vi "Dashboard Main.vi"() -> ()   [LabVIEW 2020]
uses:
  <vilib>/Utility/miscctls.llb/LVRowAndColumnTypeDef.ctl
  <vilib>/event_ctls.llb/eventvkey.ctl
  2be0e37a-cf1f-4fec-827e-dc22e69ce85b.vi
  77231be5-4dfd-47d5-a2ff-3724d3268e1c.vi
  6c3be22e-c06e-40dd-b218-0ec3cd26438d.vi
  b3ffd77c-c7a0-4f90-8868-8b56e10d7f8c.vi
  67fa5a46-adf3-4589-a2f7-66a250c43ad7.vi
  788908d1-300c-4db3-916d-f2facaeaae96.vi
  e87f41cb-5a92-4aba-b85e-f5fa50e1b7bd.vi
  bca209f3-dc8a-45d9-88b4-0d3b0861506d.vi
  fb4473b5-3a86-49a6-a9b5-0e1129129e81.vi
  849cc23d-0ef3-4264-9ef7-306e991d33d4.vi
  16c4a620-4255-445b-bb5a-a821105b922f.vi
  55761e46-cf36-4bf9-9854-b902932db1d3.vi
  <vilib>/Rock Robotics/Network Tables/NT Write Boolean.vi
  <vilib>/Rock Robotics/Network Tables/NT Read Boolean.vi
  MARS Created VIs/GlobalDataNames.vi
  <vilib>/Rock Robotics/Network Tables/NT Read Boolean Array.vi
  <vilib>/Rock Robotics/Network Tables/NT Read Numeric Array.vi
  <vilib>/Rock Robotics/Network Tables/NT Write Boolean Array.vi
  <vilib>/Rock Robotics/Network Tables/NT Write String Array.vi
  <vilib>/Rock Robotics/Network Tables/NT Write Numeric Array.vi
  <vilib>/Rock Robotics/WPI/Dashboard/WPI_DashboardLogging Global.vi
  <vilib>/Utility/Data Type/NI_Data Type.lvlib
  <vilib>/Utility/Data Type/Type Definitions/Data Type.ctl
panel:
  in  "Camera Settings":T1={"Frame Rate"=15, "Compression"=30, "Size"=1, "DB Camera Config"=TRUE} {"Frame Rate" scale=1.0..30.0; "Compression" scale=100.0..-1.0; "Size" items=["640x480", "320x240", "160x120"]}
  in  "Camera Name":string(combo)="No Camera Selection"
  out "Driver Controls":string[](array[string])=["Teleop-\nPilot-\nleft joystick X & Y axes- swerve strafe / lateral and vertical throttle (field-oriented, based on IMU)\nright joystick X axis- swerve rotational throttle\nLeft trigger- intaking balls\nLeft bumper- outtake balls\nRight trigger- fire shooter\nRight bumper- puke ball\nY button- zero pose (IMU & odometry, the odometry zeroes to touching the right post of our team’s launch pad)\nB button- disable turret safety\n\nCo-pilot-\nleft joystick X & Y- control turret field-based\nleft joystick push- change turret control to be %vbus \nright joystick Y- outer arm elevator\nleft/right bumper- inner arm pivot back/forward respectfully\nleft/right triggers- outer arm pivot back/vertical respectfully\nX button- move turret and cowl to zero\nY button- toggle climber sequence\nA button- confirm step advance\nB button- toggle always-tracking turret & passive flywheel (off by default)\nD-pad Up/Down- run magazine forwards/backwards respectfully\nD-pad right/left- run funnel forwards/backwards respectfully\n\n*the manual climb pneumatic controls only override the climb sequence when the buttons are held down. once released, the pneumatic goes back to the state it was at previously*", "Test Controls:\nPilot-\nleft joystick X & Y axes- swerve strafe / lateral and vertical throttle (robot-oriented)\nright joystick X axis- swerve rotational throttle\nA button- toggle intake pneumatic\nleft trigger- run intake motor\nRight trigger- run flywheel\nD-pad Up/Down- run magazine forwards/backwards respectfully\nD-pad right/left- run funnel forwards/backwards respectfully\nB button (hold)- disable limits on outer arm pivot, outer arm elevator, inner arm pivot, turret, and cowl\nX button- set new zero values to the current spots on those ^\nY button- zero pose (IMU & odometry)\n\nCopilot-\nleft joystick X- control turret\nright joystick Y- outer arm elevator\nleft/right bumper- inner arm pivot back/forward respectfully\nleft/right triggers- outer arm pivot back/vertical respectfully\nView/Menu button- move cowl down/up respectfully\nY button- toggle climber sequence\nA button- confirm step advance\n", "LED Colors-\nnormal\t\t\t\tred\ntargeting... \t\t\tyellow\nfiring! \t\t\t\tgreen\nno target seen\t\t\tblue\nball in magazine\t\torange\nclimb sequence started \tpurple\nclimb step finished\t\twhite\nauto is happening\t\tpink\nauto play ended\t\tbeige\n"]
  in  "TCP":refnum<k5>
  out "Robot IP":string="0.0.0.0"
  out "Image Message":string="Timeout in Camera Communications"
  in  "Dashboard Tab":T2(tab)
  in  "SWM_LL_Threshold (in)":dbl=143.0
  in  "SWM_Magnitude_Limit":dbl=0.3
  in  "SWM_Moving_Threshold (ft/s)":dbl=0.1
  in  "Turret_Max_Offset(deg)":dbl=2.0
  in  "Turret_Offset":dbl=2.0
  out "BR_Zero":dbl
  out "BR_Position":dbl
  out "BL_Zero":dbl
  out "BL_Position":dbl
  out "FL_Zero":dbl
  out "FL_Position":dbl
  out "FR_Zero":dbl
  out "FR_Position":dbl
  in  "Max_Ground_Speed(ft/s)":dbl
  in  "Cowl_Kp":dbl=0.06
  in  "Manual_Magazine_Power":dbl=0.4
  in  "Flywheel_Speed_Multiplier":dbl=1.0
  in  "Flywheel_Acceptable_Error":dbl=200.0
  in  "Turret_Upper_Limit_Value":dbl=160.0
  in  "Turret_Lower_Limit_Value":dbl=-160.0
  in  "Turret_Kd":dbl=0.001
  in  "Turret_Ki":dbl=1e-05
  in  "Turret_Kp":dbl=0.06
  in  "BL_Min Output":dbl=-0.5 min=0.0
  in  "BR_Max Ouput":dbl=0.5 min=0.0
  in  "BR_Int Error Window":dbl=20.0 min=0.0
  in  "BR_N-Int":i32=10 min=0
  in  "BR_N-Diff":i32=10 min=0
  in  "BR_Kd":dbl min=0.0
  in  "BR_Ki":dbl min=0.0
  in  "BR_Kp":dbl=0.0028 min=0.0
  in  "BL_Min Output":dbl=-0.5 min=0.0
  in  "BL_Max Ouput":dbl=0.5 min=0.0
  in  "BL_Int Error Window":dbl=20.0 min=0.0
  in  "BL_N-Int":i32=10 min=0
  in  "BL_N-Diff":i32=10 min=0
  in  "BL_Kd":dbl min=0.0
  in  "BL_Ki":dbl min=0.0
  in  "BL_Kp":dbl=0.0028 min=0.0
  in  "FL_Min Output":dbl=-0.5 min=0.0
  in  "FL_Max Ouput":dbl=0.5 min=0.0
  in  "FL_Int Error Window":dbl=20.0 min=0.0
  in  "FL_N-Int":i32=10 caption="FR_N-Int" min=0
  in  "FL_N-Diff":i32=10 min=0
  in  "FL_Kd":dbl min=0.0
  in  "FL_Ki":dbl min=0.0
  in  "FL_Kp":dbl=0.0028 min=0.0
  in  "FR_Min Output":dbl=-0.5 min=0.0
  in  "FR_Max Ouput":dbl=0.5 min=0.0
  in  "FR_Int Error Window":dbl=20.0 min=0.0
  in  "FR_N-Int":i32=10 min=0
  in  "FR_N-Diff":i32=10 min=0
  in  "FR_Kd":dbl min=0.0
  in  "FR_Ki":dbl min=0.0
  in  "FR_Kp":dbl=0.0028 min=0.0
  out "Cowl_Position(Degrees)":dbl(knob)=45.0 scale=-180.0..180.0
  out "Orientation_State":enum16{"Robot-Oriented", "Field-Oriented"}(ring)
  out "Back_Right_Drive_Command":dbl(slide) scale=0.0..1.0 scale format="%.2f"
  out "Back_Right_Angle_Command(deg)":dbl(knob) scale=180.0..-180.0 scale format="%#_6f"
  out "Back_Left_Drive_Command":dbl(slide) scale=0.0..1.0 scale format="%.2f"
  out "Back_Left_Angle_Command(deg)":dbl(knob) scale=180.0..-180.0 scale format="%#_6f"
  out "Front_Left_Drive_Command":dbl(slide) scale=0.0..1.0 scale format="%.2f"
  out "Front_Left_Angle_Command(deg)":dbl(knob) scale=180.0..-180.0 scale format="%#_6f"
  out "Front_Right_Drive_Command":dbl(slide) scale=0.0..1.0 scale format="%.2f"
  out "Front_Right_Angle_Command(deg)":dbl(knob) scale=180.0..-180.0 scale format="%#_6f"
  out "Flywheel_Velocity(RPM)":dbl(slide)=2614.0 scale=0.0..5000.0 scale format="%#_5g"
  out "Turret_Absolute_Position(Degrees)":dbl(knob)=45.0 scale=-180.0..180.0
  out "Camera Image":T3(plugin-control)
  out "Camera Perf":string="                          "
  out "Magazine_Velocity":dbl
  out "BoolTableSize":i32
  out "NumTableSize":i32
  out "StrTableSize":i32
  out "Selector":string="Initialize"
  out "NTEmpty":bool=TRUE
  out "disconnected":bool=TRUE
  out "ValuesGotOverwritten":bool
  in  "Select Auto":string(combo)="Select Autonomous ..."
  out "NT Connection":bool
  out "JS1 Z":dbl(slide) scale=-1.0..1.0 scale format="%#_2e"
  out "JS1 Graph":cluster{"X":dbl, "Y":dbl}[](graph)
  out "JS1 Buttons":T4
  out "JS2 Z":dbl(slide) scale=-1.0..1.0 scale format="%#_2e"
  out "JS2 Graph":cluster{"X":dbl, "Y":dbl}[](graph)
  out "JS2 Buttons":T4
  out "Mode":T5(ring)=enum."Disconnected"
  out "Right Camera Perf":cluster{"Bandwidth (Mbps)":dbl, "FPS":dbl}
  out "Camera Image Right":T3(plugin-control)
  in  "Camera Settings Right":T1={"Frame Rate"=15, "Compression"=30, "Size"=1, "DB Camera Config"=FALSE} {"Frame Rate" scale=1.0..30.0; "Compression" scale=100.0..-1.0; "Size" items=["640x480", "320x240", "160x120"]}
  in  "Camera Name Right":string(combo)="No Camera Selection"
  in  "Rec Mode":enum32{"Stop", "Record", "Playback"}(radio)
  in  "DB/String 9":string
  in  "DB/String 8":string
  in  "DB/String 7":string
  in  "DB/String 6":string
  in  "DB/String 5":string
  in  "DB/String 4":string
  in  "DB/String 3":string
  in  "DB/String 2":string
  in  "DB/String 1":string
  in  "DB/String 0":string
  in  "DB/Slider 0":dbl(slide) scale=0.0..5.0
  in  "DB/Slider 1":dbl(slide) scale=0.0..5.0
  in  "DB/Slider 2":dbl(slide) scale=0.0..5.0
  in  "DB/Slider 3":dbl(slide) scale=0.0..5.0
  out "DB/LED 3":bool
  out "DB/LED 2":bool
  out "DB/LED 1":bool
  out "DB/LED 0":bool
  in  "DB/Button 3":bool
  in  "DB/Button 2":bool
  in  "DB/Button 1":bool
  in  "DB/Button 0":bool caption="New Name"
  in  "Test Slider":dbl(slide) scale=0.0..100.0 scale format="%#_3g"
  in  "On/Off":bool caption="Solenoid"
  in  "Test Name":u16(ring) items=["Select the test to run..."]
  in  "Test Tree":string(tree)
  in  "Motor":cluster{"Value":dbl, "Enable":bool} {"Value" scale=-1.0..1.0 scale format="%#_3g"}
  out "Progress":T6 {"Test Progress" scale=0.0..100.0}
  in  "Rev/Fwd":cluster{"Forward":bool, "Reverse":bool}
  in  "Test Ring":u16(ring) items=["Monochrome", "Color"]
  out "Cmd Status":string
  in  "Execute Command":bool
  in  "Command Params":string[][](table)
  in  "Command Selection":i32(listbox)
  in  "CheckList":i32(listbox)
  out "Tree":string(tree)
  out "SWM_In_Range":bool
  in  "Alpha_Limelight_Mounting_Angle(deg)":dbl=35.0
  out "Limelight_Distance_To_Target (in)":dbl
  in  "Zero_Swerves":bool
  in  "Funnel_Load_%Vbus":dbl=0.7
  in  "Magazine_Load_%Vbus":dbl=0.3
  in  "Intake_Load_%Vbus":dbl=0.5
  out "Drive_IMU_Yaw":dbl
  out "Robot_Y":dbl
  out "Robot_X":dbl
  out "Limelight_Disconnected":bool
  out "Flywheel_Spun_Up":bool
  out "Turret_Locked":bool
  out "Camera Image 2":T3(plugin-control)
  in  "Auto_Play_Selector":string(combo)="A-No-Op"
  in  "Magazine_Firing_Velocity":dbl=6300.0
  out "Background":bool
  # "0- Teleop 1- Test 2- LED"
  # "HW"
  # "Funnel"
  # "Turret"
  # "Cowl"
  # "Flywheel"
  # "Constant"
  # "Magazine"
  # "Shooting While Moving"
  # "Drive"
  # "Drive Commands"
  # "Front_Left"
  # "Front_Right"
  # "Back_Left"
  # "Back_Right"
  # "Joysticks"
  # "Drive Motors"
  # "Front"
  # "Right"
  # "Left"
  # "Back"
  # "HW"
  # "This tab is a great place for autonomous settings and robot-specific values.\nPlace controls and indicators inside this tab and match name to\nDashboard Variables on robot. You can also delete this comment."
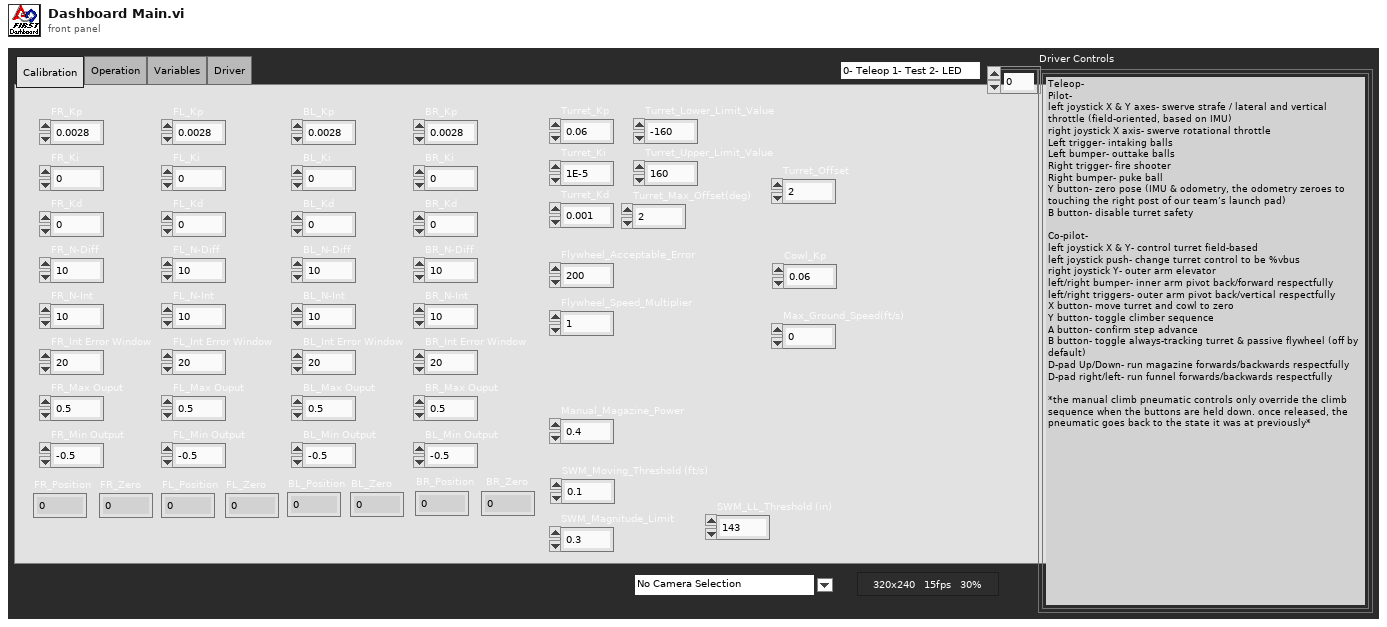
[diagram p1: front panel]
types:
  T1 = cluster{"Frame Rate":i32, "Compression":i32, "Size":u16, "DB Camera Config":bool}
  T2 = enum32{"Calibration", "Operation", "Testing", "Drive", "Camera", "Basic", "Custom", "Test", "Commands", "Checklist", "Variables", "Driver"}
  T3 = typedef "IMAQ Image.ctl" = refnum<image>
  T4 = cluster{bool, bool, bool, bool, bool, bool, bool, bool, bool, bool, bool, bool}
  T5 = enum8{"Tele-Op Disabled", "Tele-Op Enabled", "Auto Disabled", "Auto Enabled", "Test Disabled", "Test Enabled", "Disconnected", "No Code", "E-Stop"}
  T6 = cluster{"Test Progress":u8, "Test Progress Text":string}
  T7 = cluster{"Save Path":path, "Interval (s)":dbl, "Keep":i32}
  T8 = typedef "Image Type" = u32
  T9 = cluster{"IDs":cluster{"RPC field ID":u16, "Unique ID":u16}, "String":string}
  T10 = cluster{"Error Strings":string, "Disable Counts":cluster{u16, u16}, "Rail Faults":cluster{u16, u16, u16}, "Robot IP":string, "DB Mode":u8, "Event Info":cluster{"Name":string, "Type":u8, "Number":u16, "Replay":u8}}
  T11 = cluster{"Storage":cluster{"Disk Free":u64, "RAM Block":u32, "RAM free":u32}, "CPU Utilization":cluster{"CPU % ISR":sgl, "CPU % Time Crit":sgl, "CPU % Timed Str":sgl, "CPU % High":sgl, "CPU % Above":sgl, "CPU % Normal":sgl, "CPU % Low":sgl}, "CAN":cluster{"% Bus Utilization":sgl, "Bus Off Cnt":u32, "TX_FIFO Full Cnt":u32, "Receive Error Cnt":u8, "Transmit Error Cnt":u8}, "HID":cluster{"HID Outputs":u32, "Rumble Low":u16, "Rumble High":u16}[]}
  T12 = cluster{"Status bits":cluster{"Test Mode":bool, "Autonomous":bool, "Enabled":bool, "Code Start":bool, "Brownout":bool, "Reserved 2":bool, "Reserved 3":bool, "E-Stop":bool}, "Code Trace":cluster{"Disabled":bool, "TeleOp":bool, "Auto":bool, "Test":bool}, "Controller Type":enum16{"unknown", "cRIO", "roboRio"}, "Code?":enum16{"unknown", "noCode", "code"}, "Battery V":dbl}
  T13 = cluster{"Control Bits":cluster{"TestMode":bool, "Autonomous":bool, "Enabled":bool, "FMS Present":bool, bool, bool, bool, "E-Stop":bool}, "Team Station ":u8, "Countdown":sgl, "Joystick Values":cluster{"Axes":dbl[], "Buttons":bool[], "POVs":i16[]}[]}
  T14 = cluster{"Axes":dbl[], "Buttons":bool[], "POVs":i16[]}[]
  T15 = cluster{"Axes":dbl[], "Buttons":bool[], "POVs":i16[]}
  T16 = cluster{"Buttons[0]":bool, "Buttons[1]":bool, "Buttons[2]":bool, "Buttons[3]":bool, "Buttons[4]":bool, "Buttons[5]":bool, "Buttons[6]":bool, "Buttons[7]":bool, "Buttons[8]":bool, "Buttons[9]":bool, "Buttons[10]":bool, "Buttons[11]":bool}
  T17 = cluster{"Camera Image":refnum<vi>, "Dashboard Tab":refnum<vi>, "Background":refnum<vi>, "Rec Mode":refnum<vi>, "Test Slider":refnum<vi>, "On/Off ":refnum<vi>, "Test Ring":refnum<vi>, "Rev/Fwd":refnum<vi>, "Test Name":refnum<vi>, "Motor":refnum<vi>, "Progress":refnum<vi>, "CheckList":refnum<vi>, "Tree":refnum<vi>, "Test Tree":refnum<vi>, "Command Params":refnum<vi>, "Command Selection":refnum<vi>, "Execute Command":refnum<vi>, "Cmd Status":refnum<vi>, "Camera Settings":refnum<vi>, "Camera Name":refnum<vi>, "Camera Perf":refnum<vi>, "Camera Settings Right":refnum<vi>, "Camera Name Right":refnum<vi>, "Camera Image Right":refnum<vi>}
  T18 = cluster{"Global Rectangle":i32[], "Contours":cluster{"Contour Type":u32, "ROI Type":u32, "Points":i32[]}[]}
  T19 = cluster{"Camera Name":string, string, "Saved DB Images Info":cluster{"Save Path":path, "Interval (s)":dbl, "Keep":i32}}
  T20 = cluster{"Camera Name Right":string, string, "Saved DB Images Info":cluster{"Save Path":path, "Interval (s)":dbl, "Keep":i32}}
  T21 = cluster{"Operation":enum16{"Update", "Clear"}, "Color Box":u32}[]
  T22 = typedef "eventvkey.ctl" = enum16{"ASCII", "Enter", "Return", "Shift", "Ctrl", "Alt", "Cmd", "Opt", "Caps", "NumLock", "Clear", "Break", "Up", "Down", "Left", "Right", "Insert", "Delete", "Home", "End", "PageUp", "PageDown", "Escape", "Help", "Pause", "ScrollLock", "F1", "F2", "F3", "F4", "F5", "F6", "F7", "F8", "F9", "F10", "F11", "F12", "F13", "F14", "F15", "F16", "F17", "F18", "F19", "F20", "F21", "F22", "F23", "F24", "Play", "VolumeUp", "VolumeDown", "Mute", "Two Byte Char"}
  T23 = cluster{"Image Size":bool, "Image Type":bool, "Pixel Value":bool, "ROI Information":bool, "Zoom Factor":bool}
  T24 = cluster{"Operation":enum16{"Update", "Clear"}, "Color Box":u32}
  T25 = typedef "LVRowAndColumnTypeDef.ctl" = cluster{"Row":i32, "Column":i32}
  T26 = cluster{"Shift":bool, "Ctrl":bool, "Alt":bool, "Cmd":bool, "Opt":bool}
  T27 = typedef "NI_Data Type.lvlib/Data Type.ctl" = enum8{"Invalid Type", "Void", "I8", "I16", "I32", "I64", "U8", "U16", "U32", "U64", "Single Float", "Double Float", "Extended Float", "Single Complex", "Double Complex", "Extended Complex", "Enum U8", "Enum U16", "Enum U32", "Enum U64", "Single Float With Unit", "Double Float With Unit", "Extended Float With Unit", "Single Complex with Unit", "Double Complex with Unit", "Extended Complex with Unit", "Boolean", "String", "Path", "Picture", "Tag", "Array", "Cluster", "Variant", "LV Variant", "Waveform", "Timestamp", "Digital Waveform", "Digital Data", "ExpressData", "Refnum", "External Data", "VI", "Poly VI", "LabVIEW Class Instance", "Fixed Point", "Set Collection", "Map Collection"}
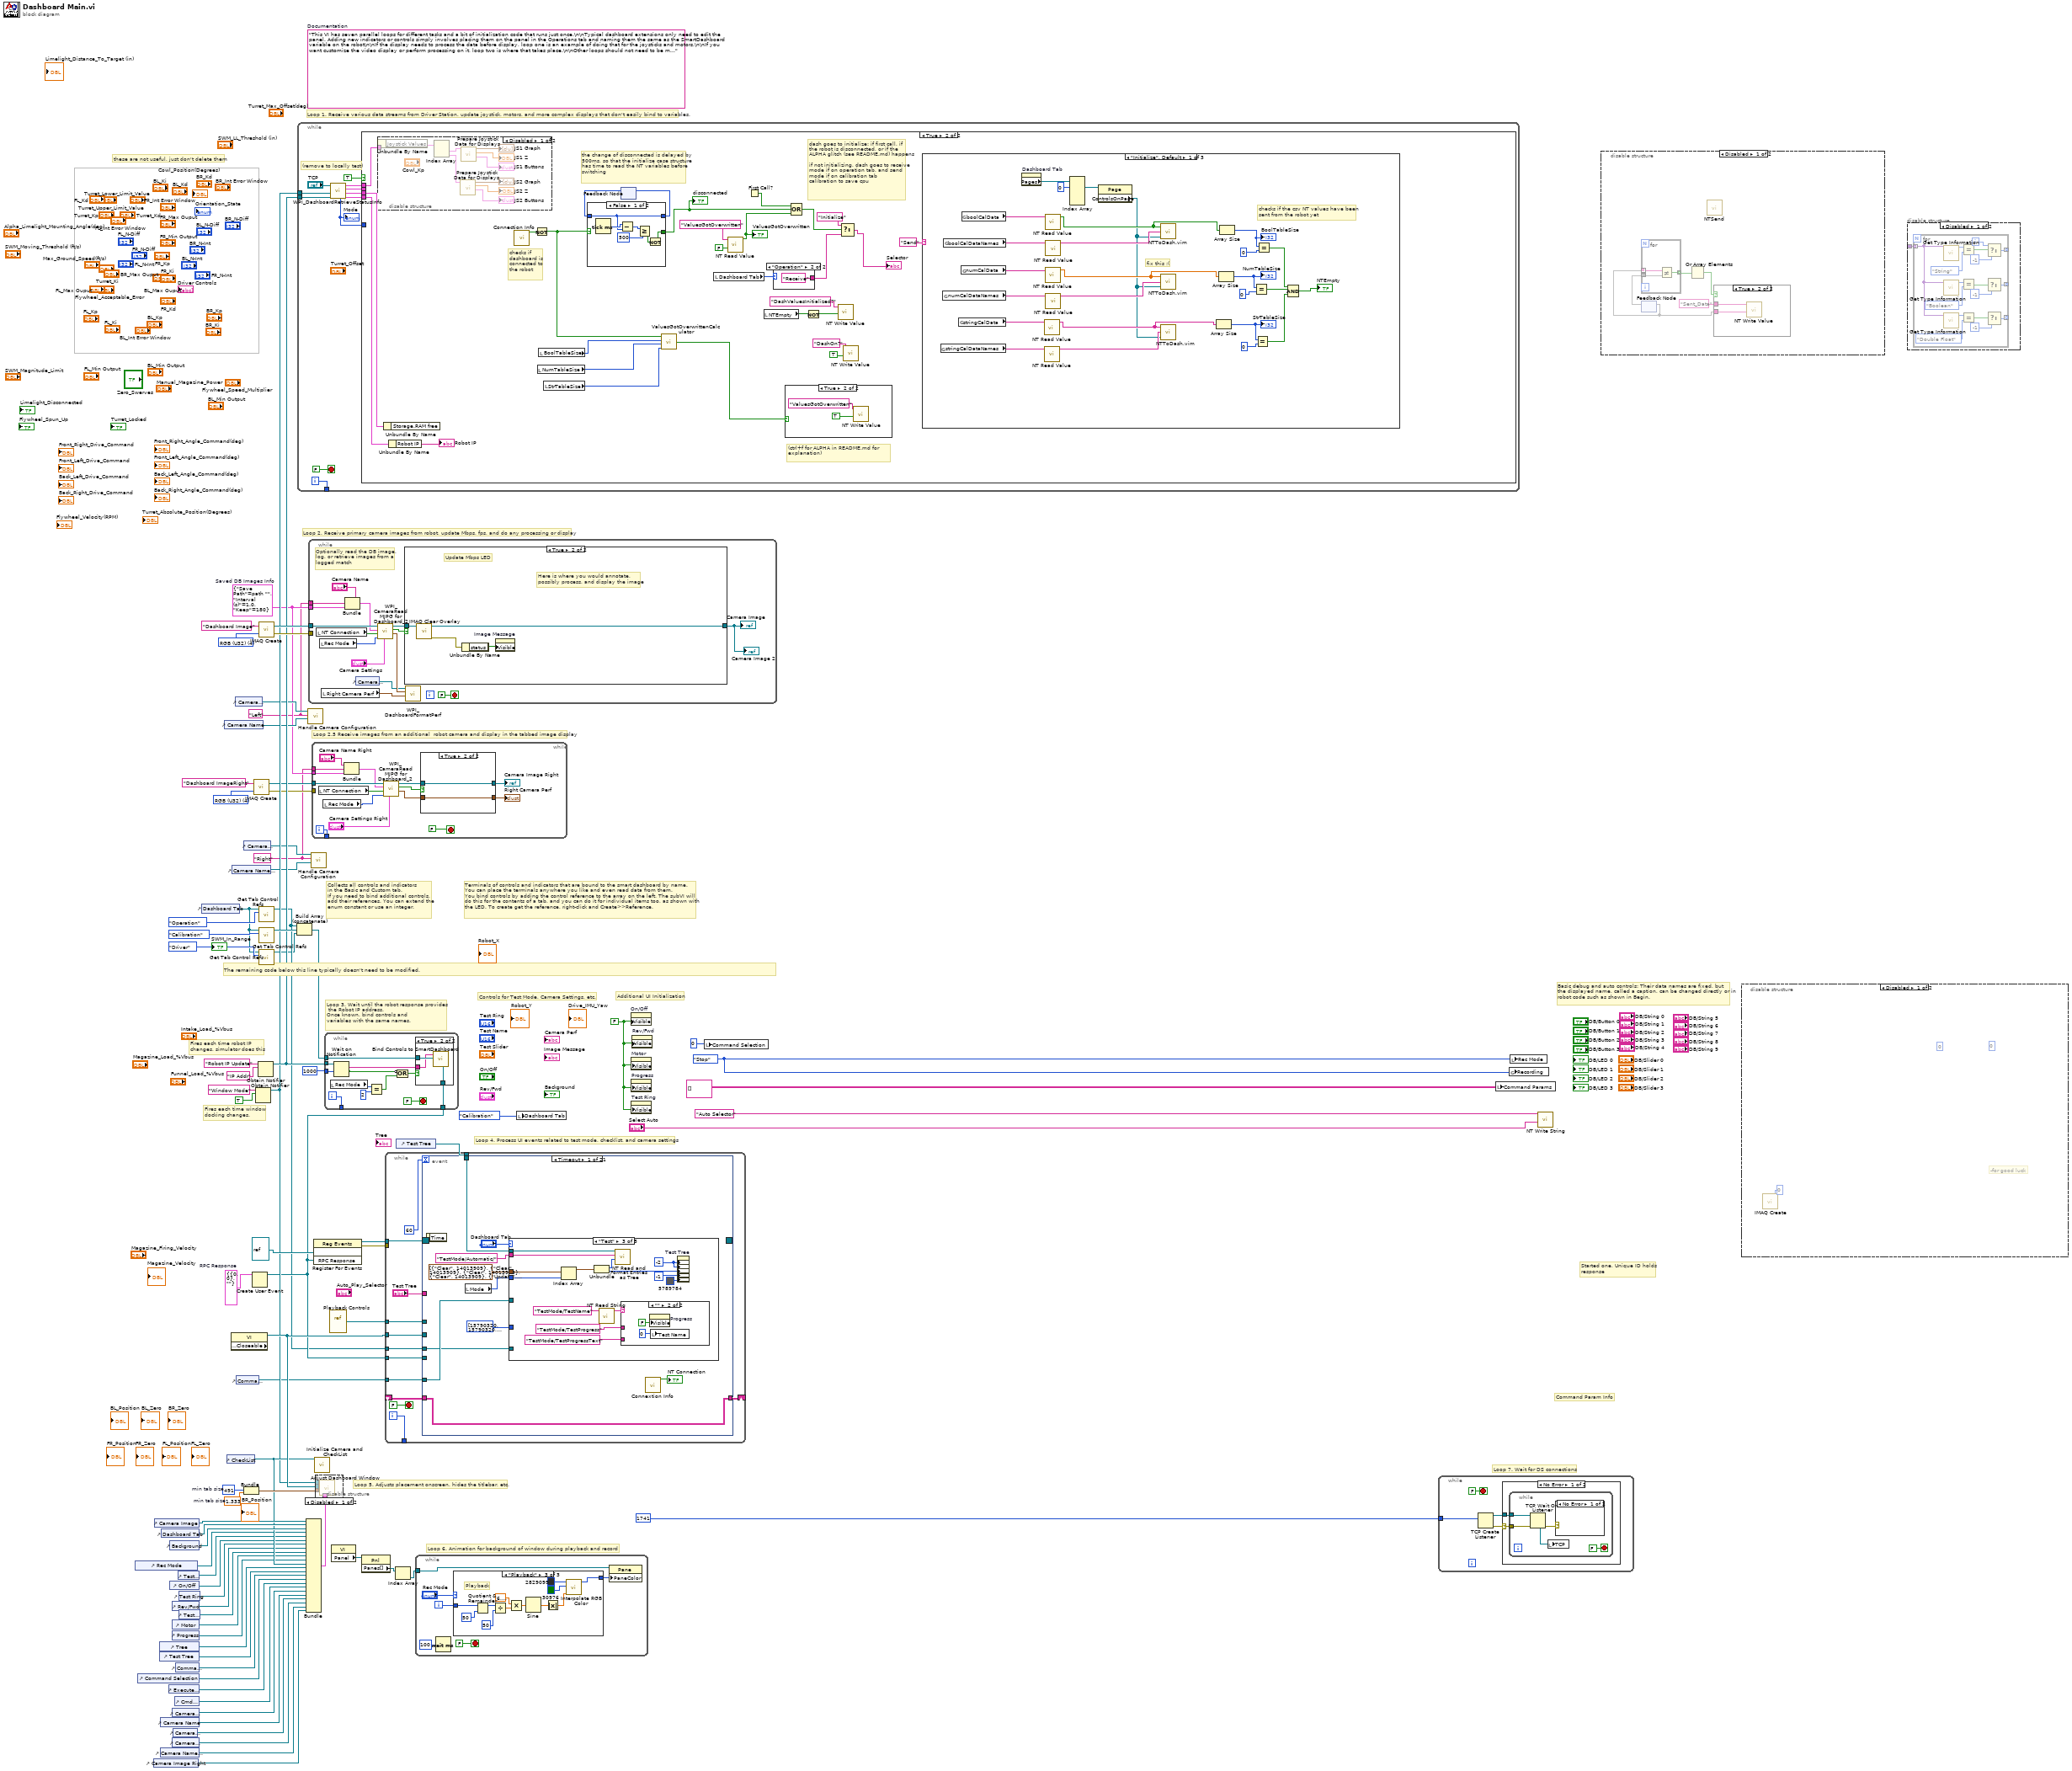
[diagram p0: block diagram]
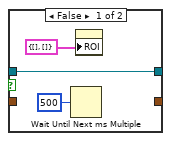
[diagram p7: hidden frame]
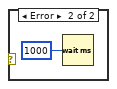
[diagram p8: hidden frame]
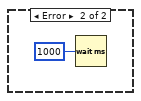
[diagram p9: hidden frame]
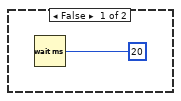
[diagram p10: hidden frame]
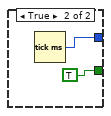
[diagram p12: hidden frame]
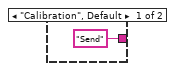
[diagram p14: hidden frame]
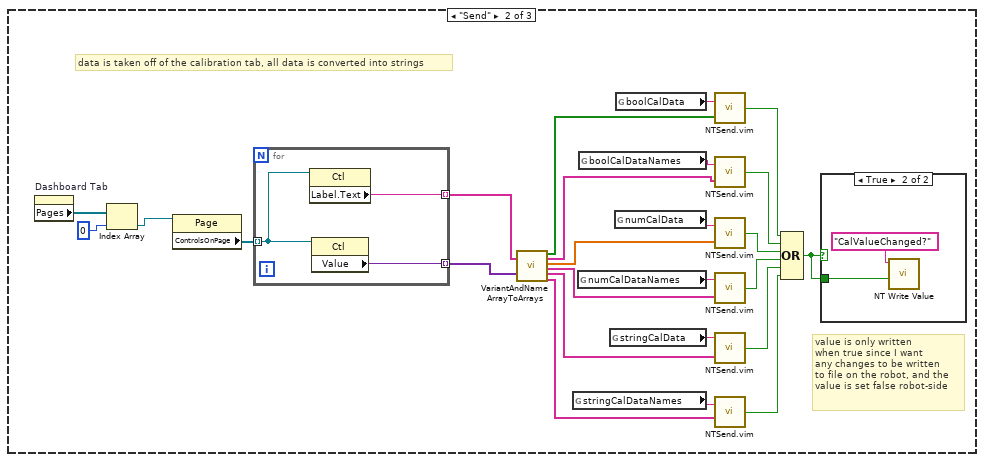
[diagram p15: hidden frame]
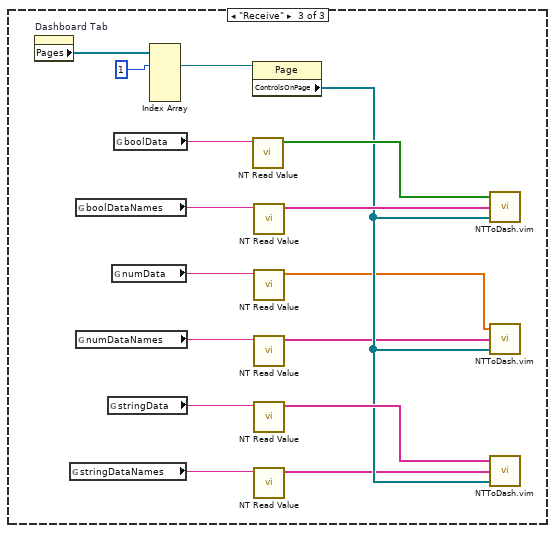
[diagram p17: hidden frame]
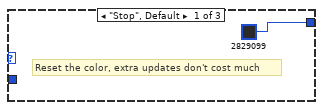
[diagram p18: hidden frame]
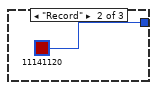
[diagram p19: hidden frame]
diagram:
  w9 = T7 {"Save Path"=path "", "Interval (s)"=1.0, "Keep"=180}  # Saved DB Images Info
  w8 = "Right"
  w7 = "Left"
  w17 = T8 4 items=["Grayscale (U8)", "Grayscale (I16)", "Grayscale (SGL)", "Complex (CSG)", "RGB (U32)", "HSL (U32)", "RGB (U64)"] ("Image Type")
  w33 = T9 {"IDs"={"RPC field ID"=0, "Unique ID"=0}, "String"=""}  # RPC Response
  w55 = 491  # min tab size
  w54 = 1.333  # min tab size
  w61 = enum32{"Stop", "Record", "Playback"}."Stop" ("Rec Mode")
  w39 = FALSE ("Visible")
  (unwired) "This VI has seven parallel loops for different tasks and a bit of initialization code that runs just once.\n\nTypical dashboard extensions only need to edit the panel. Adding new indicators or controls simply involves placing them on the panel in the Operations tab and naming them the same as the SmartDashboard variable on the robot\n\nIf the display needs to process the data before display, loop one is an example of doing that for the joysticks and motors.\n\nIf you want customize the video display or perform processing on it, loop two is where that takes place.\n\nOther loops should not need to be modified. They are pretty standard, and document the task they perform."  # Documentation
  w78 = T8 4 items=["Grayscale (U8)", "Grayscale (I16)", "Grayscale (SGL)", "Complex (CSG)", "RGB (U32)", "HSL (U32)", "RGB (U64)"] ("Image Type")
  # "these are not useful, just don't delete them"
  # "Loop 2.5 Receive images from an additional  robot camera and display in the tabbed image display"
  # "Command Param Info"
  # "Started one, Unique ID holds\nresponse"
  # "Loop 7. Wait for DS connections"
  # "Basic debug and auto controls: Their data names are fixed, but\nthe displayed name, called a caption, can be changed directly or in\nrobot code such as shown in Begin."
  # "Controls for Test Mode, Camera Settings, etc."
  # "Additional UI Initialization"
  # "Loop 6. Animation for background of window during playback and record"
  # "Fires each time robot IP\nchanges, simulator does this"
  # "Fires each time window\ndocking changes."
  # "Collects all controls and indicators\nin the Basic and Custom tab.\nIf you need to bind additional controls,\nadd their references. You can extend the\nenum constant or use an integer."
  # "The remaining code below this line typically doesn't need to be modified."
  # "Loop 4. Process UI events related to test mode, checklist, and camera settings"
  # "Terminals of controls and indicators that are bound to the smart dashboard by name.\nYou can place the terminals anywhere you like and even read data from them.\nYou bind controls by adding the control reference to the array on the left. The subVI will\ndo this for the contents of a tab, and you can do it for individual items too, as shown with\nthe LED. To create get the reference, right-click and Create>>Reference."
  # "Loop 3. Wait until the robot response provides\n the Robot IP address.\nOnce known, bind controls and\nvariables with the same names."
  # "Loop 5. Adjusts placement onscreen, hides the titlebar, etc."
  # "Loop 1. Receive various data streams from Driver Station, update joystick, motors, and more complex displays that don't easily bind to variables."
  # "Loop 2. Receive primary camera images from robot, update Mbps, fps, and do any processing or display"
  n1 = control-ref of="Rec Mode"() -> (w45:refnum<vi>)
  n2 = control-ref of="Command Selection"() -> (w32:refnum<vi>)
  n3 = control-ref of="Camera Image Right"() -> (w10:refnum<vi>)
  n4 = control-ref of="Camera Image"() -> (w57:refnum<vi>)
  n5 = control-ref of="Tree"() -> (w49:refnum<vi>)
  n6 = control-ref of="Test Tree"() -> (w48:refnum<vi>)
  n7 = control-ref of="Camera Name"() -> (w23:refnum<vi>)
  n8 = control-ref of="Camera Name Right"() -> (w11:refnum<vi>)
  n9 = control-ref of="Dashboard Tab"() -> (w56:refnum<vi>)
  n10 = control-ref of="Execute Command"() -> (w34:refnum<vi>)
  n11 = control-ref of="Background"() -> (w52:refnum<vi>)
  n12 = control-ref of="On/Off"() -> (w43:refnum<vi>)
  n13 = control-ref of="Progress"() -> (w40:refnum<vi>)
  n14 = control-ref of="Camera Settings"() -> (w24:refnum<vi>)
  n15 = control-ref of="Camera Settings Right"() -> (w12:refnum<vi>)
  n16 = control-ref of="Rev/Fwd"() -> (w41:refnum<vi>)
  n17 = control-ref of="Motor"() -> (w46:refnum<vi>)
  n18 = control-ref of="Camera Perf"() -> (w22:refnum<vi>)
  n19 = control-ref of="Cmd Status"() -> (w28:refnum<vi>)
  n20 = control-ref of="Command Params"() -> (w35:refnum<vi>)
  n21 = control-ref of="Test Slider"() -> (w44:refnum<vi>)
  n22 = control-ref of="Test Ring"() -> (w42:refnum<vi>)
  n23 = control-ref of="Test Name"() -> (w47:refnum<vi>)
  n24 = control-ref of="Dashboard Tab"() -> (w2:refnum<vi>)
  n25 = control-ref of="Camera Name"() -> (w25:refnum<vi>)
  n26 = control-ref of="CheckList"() -> (w50:refnum<vi>)
  n27 = property class="VI" props=["Front Panel.Closeable"]() -> (reference out=w60:refnum<vi>)  [unwired: 2 in, 2 out]
  n28 = control-ref of="Camera Name Right"() -> (w13:refnum<vi>)
  n29 = control-ref of="Camera Settings"() -> (w26:refnum<vi>)
  n30 = control-ref of="Command Params"() -> (w27:refnum<vi>)
  n31 = control-ref of="Camera Settings Right"() -> (w14:refnum<vi>)
  n32 = Bundle("min tab size"=w55, "min tab size"=w54) -> (w53:cluster{"min tab size":i32, "min tab size":dbl})  [unwired: 1 in]
  n33 = Create User Event(user event datatype=w33) -> (user event=w29:refnum<user-event>)  [unwired: 1 in, 1 out]
  n34 = call "IMAQ Create"("Image Name"="Dashboard ImageRight", "Image Type"=w17) -> ("New Image"=w16:T3, "error out"=w15:errorcluster)  [unwired: 2 in, 1 out]
  n35 = Obtain Notifier(name (unnamed)="Window Mode", notification data type=TRUE) -> (notifier out=w37:refnum<notifier>)  [unwired: 2 in, 2 out]
  n36 = Obtain Notifier(name (unnamed)="Robot IP Update", notification data type="IP Addr" ("name (unnamed)")) -> (notifier out=w38:refnum<notifier>)  [unwired: 2 in, 2 out]
  n37 = call "IMAQ Create"("Image Name"="Dashboard Image", "Image Type"=w78) -> ("New Image"=w76:T3, "error out"=w75:errorcluster)  [unwired: 2 in, 1 out]
  n38 = call <vilib>:"Get Tab Control Refs.vi"("Page Index"=T2."Operation" ("Dashboard Tab"), "TabControl in"=w2) -> ("ControlsOnPage"=w21:refnum<vi>[])  [unwired: 9 in]
  n39 = call <vilib>:"Get Tab Control Refs.vi"("Page Index"=T2."Calibration" ("Dashboard Tab"), "TabControl in"=w2) -> ("ControlsOnPage"=w59:refnum<vi>[])  [unwired: 9 in]
  n40 = call <vilib>:"Get Tab Control Refs.vi"("Page Index"=T2."Driver" ("Dashboard Tab"), "TabControl in"=w2) -> ("ControlsOnPage"=w4:refnum<vi>[])  [unwired: 9 in]
  n41 = Build Array (concatenate)(w21, w59, w4) -> (w58:refnum<vi>[])
  n42 = while {
    tunnel: [w88] -> _
    tunnel: w38 -> [w83]
    tunnel: w37 -> [w80]
    i -> [w88]
    stop <- FALSE stop-if-true
    # "(remove to locally test)"
    n43 = call <vilib>:"WPI_DashboardRetrieveStatusInfo.vi"("Binding Refnum"=w83, "Window Mode Notifier"=w80, "TCP Cnx"="TCP") -> ("Power and Errors"=w84:T10, "Robot Metrics"=w86:T11, "Status Info"=w87:T12, "Control Info"=w85:T13, "Robot Mode"=w82:T5)  [unwired: 3 in, 1 out]
    "Mode" <- w82
    n44 = case shown="True" TRUE {
      tunnel: w87 -> [_ _]
      tunnel: w86 -> [_ w118]
      tunnel: w85 -> [_ w117]
      tunnel: w84 -> [_ w116]
      tunnel: w82 -> [_ _]
      frame False {
        n45 = Wait (ms)(milliseconds to wait=u32 20) -> ()  [unwired: 1 out]
      }
      frame True {
        # "checks if dashboard is connected to the robot"
        # "(ctrl+f for ALPHA in README.md for explanation)"
        # "the change of disconnected is delayed by 500ms, so that the initialize case structure has time to read the NT variables before switching"
        # "dash goes to initialize: if first call, if\nthe robot is disconnected, or if the ALPHA glitch (see README.md) happens\n\nif not initializing, dash goes to receive mode if on operation tab, and send mode if on calibration tab\ncalibration to save cpu"
        n46 = disable-structure shown="Disabled" {
          disable-tunnel: w117 -> [w138 _]
          frame Disabled {
            n47 = Unbundle By Name(w138) -> ("Joystick Values"=w137:T14)
            n48 = Index Array(array=w137) -> (element #1=w136:T15, element #2=w132:T15)  [unwired: 2 in]
            n49 = call "Prepare Joystick Data for Displays.vi"("Joystick Values"=w132) -> ("Buttons"=→"JS2 Buttons":T16, "Z Axis"=→"JS2 Z":dbl, "Cartesian Data"=→"JS2 Graph":cluster{"X axis":dbl, "X axis":dbl}[])  [unwired: 8 in]
            n50 = call "Prepare Joystick Data for Displays.vi"("Joystick Values"=w136) -> ("Buttons"=→"JS1 Buttons":T16, "Z Axis"=→"JS1 Z":dbl, "Cartesian Data"=→"JS1 Graph":cluster{"X axis":dbl, "X axis":dbl}[])  [unwired: 8 in]
          }
          frame Enabled {
          }
        }
        n51 = Unbundle By Name(w118) -> ()  [unwired: 1 out]
        n52 = Unbundle By Name(w116) -> ("Robot IP"=→"Robot IP":string)
        n53 = call <vilib>:"Connection Info.vi"() -> ("Connected"=w104:bool)  [unwired: 10 in, 1 out]
        n54 = Not(x=w104) -> (.not. x?=w97:bool)
        n55 = local read "NumTableSize"() -> (w99:i32)
        n56 = local read "BoolTableSize"() -> (w100:i32)
        n57 = local read "StrTableSize"() -> (w98:i32)
        n58 = feedback #1() -> (w101:u32)  [unwired: 1 in]
        n59 = case shown="False" w97 {
          tunnel: [w121 TRUE] -> w103
          tunnel: [w125 w127] -> w102
          tunnel: w101 -> [w125 _]
          frame False {
            n60 = Tick Count (ms)() -> (millisecond timer value=w126:u32)
            n61 = Subtract(x=w126, y=w125) -> (x-y=w124:u32)
            n62 = Greater Or Equal?(x=w124, y=u32 500) -> (x >= y?=w122:bool)
            n63 = Not(x=w122) -> (.not. x?=w121:bool)
          }
          frame True {
            n64 = Tick Count (ms)() -> (millisecond timer value=w127:u32)
          }
        }
        "disconnected" <- w103
        n65 = feedback-in #1(w102) -> ()
        n66 = call "ValuesGotOverwrittenCalculator.vi"("StrTableSize"=w98, "NumTableSize"=w99, "BoolTableSize"=w100, "disconnected"=w97) -> ("ValuesGotOverwritten"=w96:bool)
        n67 = local read "Dashboard Tab"() -> (w112:T2)
        n68 = call-poly <vilib>:"NT Read Value.vi"("Default Value"=FALSE, "Name"="ValuesGotOverwritten") -> ("Boolean"=w93:bool)  [unwired: 8 in, 1 out]
        "ValuesGotOverwritten" <- w93
        n69 = First Call?() -> (First Call?: T/F=w105:bool)
        n70 = local read "NTEmpty"() -> (w107:bool)
        n71 = case shown="\"Operation\"" w112 {
          tunnel: ["Send" "Receive"] -> w111
          frame "Calibration", Default {
          }
          frame "Operation" {
          }
        }
        n72 = case shown="True" w96 {
          frame False {
          }
          frame True {
            n73 = call-poly <vilib>:"NT Write Value.vi"("Boolean"=TRUE, "Name"="ValuesGotOverwritten") -> ()  [unwired: 9 in, 1 out]
          }
        }
        n74 = Compound Arithmetic op=OR(w105, w103, w93) -> (w109:bool)
        n75 = Not(x=w107) -> (.not. x?=w106:bool)
        n76 = call-poly <vilib>:"NT Write Value.vi"("Boolean"=w106, "Name"="DashValuesInitialized?") -> ()  [unwired: 9 in, 1 out]
        n77 = Select(t="Initialize", s=w109, f=w111) -> (s? t:f=→"Selector":string)
        n78 = call-poly <vilib>:"NT Write Value.vi"("Boolean"=TRUE, "Name"="DashOn?") -> ()  [unwired: 9 in, 1 out]
        n79 = case shown="\"Initialize\", Default" "Send" ("s? t:f") {
          frame "Initialize", Default {
            # "fix this :("
            # "checks if the csv NT values have been\nsent from the robot yet"
            n80 = global read "GlobalDataNames.vi" "stringCalDataNames"() -> (w155:string)
            n81 = global read "GlobalDataNames.vi" "numCalDataNames"() -> (w157:string)
            n82 = global read "GlobalDataNames.vi" "boolCalDataNames"() -> (w160:string)
            n83 = global read "GlobalDataNames.vi" "stringCalData"() -> (w156:string)
            n84 = global read "GlobalDataNames.vi" "numCalData"() -> (w158:string)
            n85 = global read "GlobalDataNames.vi" "boolCalData"() -> (w159:string)
            n86 = property on="Dashboard Tab" class="TabCtl (strict)"() -> ("Pages"=w161:refnum<vi>[])  [unwired: 2 in, 2 out]
            n87 = call-poly <vilib>:"NT Read Value.vi"("Name"=w156) -> ("String Array"=w153:string[])  [unwired: 9 in, 1 out]
            n88 = call-poly <vilib>:"NT Read Value.vi"("Name"=w155) -> ("String Array"=w165:string[])  [unwired: 9 in, 1 out]
            n89 = call-poly <vilib>:"NT Read Value.vi"("Name"=w159) -> ("Boolean Array"=w154:bool[])  [unwired: 9 in, 1 out]
            n90 = call-poly <vilib>:"NT Read Value.vi"("Name"=w158) -> ("Numeric Array"=w142:dbl[])  [unwired: 9 in, 1 out]
            n91 = call-poly <vilib>:"NT Read Value.vi"("Name"=w160) -> ("String Array"=w166:string[])  [unwired: 9 in, 1 out]
            n92 = call-poly <vilib>:"NT Read Value.vi"("Name"=w157) -> ("String Array"=w164:string[])  [unwired: 9 in, 1 out]
            n93 = Index Array(array=w161, index #1=0 ("index")) -> (element #1=w163:refnum<vi>)  [unwired: 4 in, 4 out]
            n94 = property class="Page"(reference=w163) -> ("ControlsOnPage"=w141:refnum<vi>[])  [unwired: 1 in, 2 out]
            n95 = call "NTToDash.vim"("Controls on Page[]"=w141, "Names Array"=w166, "Data Array"=w154) -> ()  [unwired: 1 in]
            n96 = call "NTToDash.vim"("Controls on Page[]"=w141, "Names Array"=w164, "Data Array"=w142) -> ()  [unwired: 1 in]
            n97 = call "NTToDash.vim"("Controls on Page[]"=w141, "Names Array"=w165, "Data Array"=w153) -> ()  [unwired: 1 in]
            n98 = Array Size(array=w153) -> (size(s)=w148:i32)
            "StrTableSize" <- w148
            n99 = Array Size(array=w142) -> (size(s)=w150:i32)
            "NumTableSize" <- w150
            n100 = Array Size(array=w154) -> (size(s)=w152:i32)
            "BoolTableSize" <- w152
            n101 = Equal?(x=w150, y=0 ("size(s)")) -> (x = y?=w145:bool)
            n102 = Equal?(x=w148, y=0 ("size(s)")) -> (x = y?=w146:bool)
            n103 = Equal?(x=w152, y=0 ("size(s)")) -> (x = y?=w144:bool)
            n104 = Compound Arithmetic op=AND(w144, w145, w146) -> (→"NTEmpty":bool)
          }
          frame "Send" {
            # "value is only written\nwhen true since I want\nany changes to be written\nto file on the robot, and the \nvalue is set false robot-side"
            # "data is taken off of the calibration tab, all data is converted into strings"
            n105 = property on="Dashboard Tab" class="TabCtl (strict)"() -> ("Pages"=w191:refnum<vi>[])  [unwired: 2 in, 2 out]
            n106 = Index Array(array=w191, index=0) -> (element=w189:refnum<vi>)
            n107 = property class="Page"(reference=w189) -> ("ControlsOnPage"=w188:refnum<vi>[])  [unwired: 1 in, 2 out]
            n108 = for {
              tunnel: w188 -> [w196] mode=indexing
              tunnel: [w195] -> w187 mode=indexing
              tunnel: [w194] -> w186 mode=indexing
              n109 = property class="Ctl"(reference=w196) -> ("Label.Text"=w195:string)  [unwired: 1 in, 2 out]
              n110 = property class="Ctl"(reference=w196) -> ("Value"=w194:variant)  [unwired: 1 in, 2 out]
            }
            n111 = call "VariantAndNameArrayToArrays.vi"("Names Array"=w187, "Variant Array"=w186) -> ("bool"=w185:bool[], "boolNames"=w184:string[], "num"=w182:dbl[], "numNames"=w181:string[], "string"=w167:string[], "stringNames"=w183:string[])  [unwired: 12 in]
            n112 = global read "GlobalDataNames.vi" "stringCalDataNames"() -> (w176:string)
            n113 = global read "GlobalDataNames.vi" "numCalDataNames"() -> (w178:string)
            n114 = global read "GlobalDataNames.vi" "boolCalDataNames"() -> (w179:string)
            n115 = global read "GlobalDataNames.vi" "stringCalData"() -> (w177:string)
            n116 = global read "GlobalDataNames.vi" "numCalData"() -> (w180:string)
            n117 = global read "GlobalDataNames.vi" "boolCalData"() -> (w175:string)
            n118 = call "NTSend.vim"("Array"=w185, "name"=w175) -> ("Write?"=w174:bool)
            n119 = call "NTSend.vim"("Array"=w184, "name"=w179) -> ("Write?"=w173:bool)
            n120 = call "NTSend.vim"("Array"=w182, "name"=w180) -> ("Write?"=w172:bool)
            n121 = call "NTSend.vim"("Array"=w181, "name"=w178) -> ("Write?"=w171:bool)
            n122 = call "NTSend.vim"("Array"=w167, "name"=w177) -> ("Write?"=w170:bool)
            n123 = call "NTSend.vim"("Array"=w183, "name"=w176) -> ("Write?"=w169:bool)
            n124 = Compound Arithmetic op=OR(w174, w173, w172, w171, w170, w169) -> (w168:bool)
            n125 = case shown="True" w168 {
              tunnel: w168 -> [_ w193]
              frame False {
              }
              frame True {
                n126 = call-poly <vilib>:"NT Write Value.vi"("Boolean"=w193, "Name"="CalValueChanged?") -> ()  [unwired: 9 in, 1 out]
              }
            }
          }
          frame "Receive" {
            n127 = property on="Dashboard Tab" class="TabCtl (strict)"() -> ("Pages"=w210:refnum<vi>[])  [unwired: 2 in, 2 out]
            n128 = global read "GlobalDataNames.vi" "stringDataNames"() -> (w204:string)
            n129 = global read "GlobalDataNames.vi" "boolDataNames"() -> (w209:string)
            n130 = global read "GlobalDataNames.vi" "numDataNames"() -> (w206:string)
            n131 = global read "GlobalDataNames.vi" "stringData"() -> (w205:string)
            n132 = global read "GlobalDataNames.vi" "numData"() -> (w207:string)
            n133 = global read "GlobalDataNames.vi" "boolData"() -> (w208:string)
            n134 = Index Array(array=w210, index #1=1 ("index")) -> (element #1=w212:refnum<vi>)  [unwired: 4 in, 4 out]
            n135 = property class="Page"(reference=w212) -> ("ControlsOnPage"=w200:refnum<vi>[])  [unwired: 1 in, 2 out]
            n136 = call-poly <vilib>:"NT Read Value.vi"("Name"=w208) -> ("Boolean Array"=w203:bool[])  [unwired: 9 in, 1 out]
            n137 = call-poly <vilib>:"NT Read Value.vi"("Name"=w209) -> ("String Array"=w202:string[])  [unwired: 9 in, 1 out]
            n138 = call-poly <vilib>:"NT Read Value.vi"("Name"=w207) -> ("Numeric Array"=w198:dbl[])  [unwired: 9 in, 1 out]
            n139 = call-poly <vilib>:"NT Read Value.vi"("Name"=w206) -> ("String Array"=w197:string[])  [unwired: 9 in, 1 out]
            n140 = call-poly <vilib>:"NT Read Value.vi"("Name"=w205) -> ("String Array"=w201:string[])  [unwired: 9 in, 1 out]
            n141 = call-poly <vilib>:"NT Read Value.vi"("Name"=w204) -> ("String Array"=w199:string[])  [unwired: 9 in, 1 out]
            n142 = call "NTToDash.vim"("Controls on Page[]"=w200, "Names Array"=w202, "Data Array"=w203) -> ()  [unwired: 1 in]
            n143 = call "NTToDash.vim"("Controls on Page[]"=w200, "Names Array"=w197, "Data Array"=w198) -> ()  [unwired: 1 in]
            n144 = call "NTToDash.vim"("Controls on Page[]"=w200, "Names Array"=w199, "Data Array"=w201) -> ()  [unwired: 1 in]
          }
        }
      }
    }
  }
  n145 = Bundle("Camera Image"=w57, "Dashboard Tab"=w56, "Background"=w52, "Rec Mode"=w45, "Test Slider"=w44, "On/Off"=w43, "Test Ring"=w42, "Rev/Fwd"=w41, "Test Name"=w47, "Motor"=w46, "Progress"=w40, "CheckList"=w50, "Tree"=w49, "Test Tree"=w48, "Command Params"=w35, "Command Selection"=w32, "Execute Command"=w34, "Cmd Status"=w28, "Camera Settings"=w24, "Camera Name"=w23, "Camera Perf"=w22, "Camera Settings Right"=w12, "Camera Name Right"=w11, "Camera Image Right"=w10) -> (w51:T17)  [unwired: 1 in]
  n146 = call "Handle Camera Configuration.vi"("CameraNameRef"=w25, "Display Name"=w7, "ClusterRef"=w26) -> ()  [unwired: 9 in]
  n147 = while {
    tunnel: w76 -> [w226]
    tunnel: w75 -> [_]
    tunnel: w9 -> [w220]
    tunnel: w7 -> [w217]
    stop <- FALSE stop-if-true
    # "Optionally read the DB image,\nlog, or retrieve images from a\nlogged match"
    n148 = local read "NT Connection"() -> (w221:bool)
    n149 = local read "Rec Mode"() -> (w223:enum32{"Stop", "Record", "Playback"})
    n150 = local read "Right Camera Perf"() -> (w215:cluster{"Bandwidth (Mbps)":dbl, "FPS":dbl})
    n151 = Bundle("Camera Name"="Camera Name", w217, "Saved DB Images Info"=w220) -> (w219:T19)  [unwired: 1 in]
    n152 = control-ref of="Camera Perf"() -> (w214:refnum<vi>)
    n153 = call <vilib>:"WPI_CameraRead MJPG for Dashboard_2.vi"("Camera Settings"="Camera Settings", "Rec Mode"=w223, "NT Connection"=w221, "Capture Info"=w219, "Image in"=w226) -> ("perf info"=w216:cluster{"Bandwidth (Mbps)":dbl, "fps":dbl}, "Active"=w224:bool, "Image\\ out"=w225:T3)  [unwired: 4 in]
    n154 = case shown="True" w224 {
      tunnel: w225 -> [w229 w232]
      tunnel: [w229 w231] -> w213
      frame False {
        # "Sleep for 500ms"
        n155 = property on="Camera Image" class="ImageControl"("ROI"=T18 {"Global Rectangle"=[], "Contours"=[]}) -> ()  [unwired: 2 in, 2 out]
        n156 = Wait Until Next ms Multiple(millisecond multiple=u32 500) -> ()  [unwired: 1 out]
      }
      frame True {
        # "Here is where you would annotate,\npossibly process, and display the image"
        # "Update Mbps LED"
        n157 = call "IMAQ Clear Overlay"("Image"=w232) -> ("error out"=w233:errorcluster, "Image Out"=w231:T3)  [unwired: 2 in, 7 out]
        n158 = Unbundle By Name(w233) -> ("status"=w234:bool)
        n159 = property on="Image Message" class="Str"("Visible"=w234) -> ()  [unwired: 2 in, 2 out]
      }
    }
    "Camera Image" <- w213
    "Camera Image 2" <- w213
    n160 = call <vilib>:"WPI_DashboardFormatPerf.vi"("Right Camera Perf"=w215, "Performance"=w216, "String in"=w214) -> ()  [unwired: 9 in]
  }
  n161 = call "Handle Camera Configuration.vi"("CameraNameRef"=w13, "Display Name"=w8, "ClusterRef"=w14) -> ()  [unwired: 9 in]
  n162 = while {
    tunnel: w16 -> [w249]
    tunnel: w15 -> [_]
    tunnel: [w244] -> _
    tunnel: w9 -> [w240]
    tunnel: w8 -> [w237]
    i -> [w244]
    stop <- FALSE stop-if-true
    n163 = local read "NT Connection"() -> (w241:bool)
    n164 = local read "Rec Mode"() -> (w248:enum32{"Stop", "Record", "Playback"})
    n165 = Bundle("Camera Name Right"="Camera Name Right", w237, "Saved DB Images Info"=w240) -> (w239:T20)  [unwired: 1 in]
    n166 = call <vilib>:"WPI_CameraRead MJPG for Dashboard_2.vi"("Camera Settings"="Camera Settings Right", "Rec Mode"=w248, "NT Connection"=w241, "Capture Info"=w239, "Image in"=w249) -> ("perf info"=w235:cluster{"Bandwidth (Mbps)":dbl, "fps":dbl}, "Active"=w243:bool, "Image\\ out"=w246:T3)  [unwired: 4 in]
    n167 = case shown="True" w243 {
      tunnel: w246 -> [w251 w254]
      tunnel: [w251 w254] -> w242
      tunnel: [_ w253] -> w236
      tunnel: w235 -> [_ w253]
      frame False {
        n168 = Wait Until Next ms Multiple(millisecond multiple=u32 500) -> ()  [unwired: 1 out]
        n169 = property on="Camera Image Right" class="ImageControl"("ROI"=T18 {"Global Rectangle"=[], "Contours"=[]}) -> ()  [unwired: 2 in, 2 out]
      }
      frame True {
      }
    }
    "Camera Image Right" <- w242
    "Right Camera Perf" <- w236
  }
  n170 = register-events(refnum<vi> refnum, w29) -> (reference out=w65:refnum<event-registration>, error out=w64:errorcluster)  [unwired: 2 in]
  n171 = call "Initialize Camera and CheckList.vi"("ListBox in"=w50) -> ()  [unwired: 11 in]
  n172 = disable-structure shown="Disabled" {
    disable-tunnel: w60 -> [w258 _]
    disable-tunnel: w53 -> [w257 _]
    disable-tunnel: w51 -> [w256 _]
    disable-tunnel: w37 -> [w255 _]
    frame Disabled {
      n173 = call "Adjust Dashboard Window.vi"("Sizing Refnums"=w256, "Size Constraints"=w257, "VI"=w258, "WIn Mode"=w255) -> ()  [unwired: 8 in]
    }
    frame Enabled {
    }
  }
  n174 = while {
    tunnel: w58 -> [w270]
    tunnel: w38 -> [w268]
    tunnel: [w266] -> _
    tunnel: u32 1000 ("milliseconds to wait") -> [w265]
    tunnel: w29 -> [w259]
    i -> [w266]
    stop <- FALSE stop-if-true
    n175 = local read "Rec Mode"() -> (w261:enum32{"Stop", "Record", "Playback"})
    n176 = Wait on Notification(notifier=w268, timeout in ms (-1)=w265) -> (notification=w267:string, timed out?=w263:bool)  [unwired: 2 in, 2 out]
    n177 = Equal?(x=w261, y=u16 2 ("Rec Mode")) -> (x = y?=w262:bool)
    n178 = Compound Arithmetic op=OR(invert w263, w262) -> (w264:bool)
    n179 = case shown="True" w264 {
      tunnel: w270 -> [_ w273]
      tunnel: w267 -> [_ w272]
      tunnel: w259 -> [_ w271]
      frame False {
      }
      frame True {
        n180 = call <vilib>:"Bind Controls to SmartDashboard.vi"("RPC ref"=w271, "Bound Control Refs"=w273, "Server IP Address"=w272) -> ()  [unwired: 9 in]
      }
    }
  }
  n181 = vi-ref "Playback Controls.vi"() -> (w66:refnum<vi>)
  n182 = property class="VI"() -> ("Panel"=w68:refnum<vi>)  [unwired: 2 in, 2 out]
  n183 = property class="Pnl"(reference=w68) -> ("Panes[]"=w69:refnum<vi>[])  [unwired: 1 in, 2 out]
  n184 = Index Array(array=w69) -> (element=w67:refnum<vi>)  [unwired: 1 in]
  n185 = control-ref of="Test Tree"() -> (w70:refnum<vi>)
  n186 = while {
    tunnel: [w283] -> _
    tunnel: w70 -> [w282]
    tunnel: w66 -> [w281]
    tunnel: w65 -> [w280]
    tunnel: w64 -> [_]
    tunnel: w60 -> [w279]
    tunnel: w29 -> [w278]
    tunnel: w27 -> [w277]
    shift-right: [w276] -> _
    shift-left: _ -> [w275]
    tunnel: w21 -> [w274]
    i -> [w283]
    stop <- FALSE stop-if-true
    n187 = event shown="[0] Timeout" {
      selector: w280 -> [_ _ _ _ _ _ _ _ _ _ _ _ _ _ _ _ _ _ _ _ _]
      dyn-events: [_ _ _ _ _ _ _ _ _ _ _ _ _ _ _ _ w543 _ _ _ _] -> _
      timeout: u32 60 ("milliseconds to wait") -> [_ _ _ _ _ _ _ _ _ _ _ _ _ _ _ _ _ _ _ _ _]
      tunnel: w282 -> [w295 _ _ _ _ _ _ _ _ _ _ _ _ _ _ _ _ _ _ _ _]
      tunnel: "Test Tree" -> [_ _ _ _ _ _ _ _ _ _ _ w510 w518 w520 w524 w532 _ _ _ _ _]
      tunnel: w281 -> [_ _ _ _ _ _ _ _ _ _ _ _ _ _ _ _ w545 _ w563 _ _]
      tunnel: w279 -> [_ _ _ _ _ _ _ _ _ _ _ _ _ _ _ _ w541 _ _ _ _]
      tunnel: w278 -> [_ _ _ _ _ _ _ _ _ _ _ _ _ _ _ _ w539 _ _ _ _]
      tunnel: w277 -> [w290 _ _ _ _ _ w461 _ _ _ _ _ _ _ _ _ _ _ _ _ _]
      tunnel: [w289 w338 w440 w445 w454 w458 w459 w468 w478 w485 w497 w509 w516 w519 w523 w531 w538 w558 w560 w564 w577] -> w276
      tunnel: w275 -> [w289 w338 w440 w445 w454 w458 w459 _ _ w485 w497 w509 w516 w519 w523 w531 w538 w558 w560 w564 w577]
      tunnel: w274 -> [w287 _ _ _ _ _ _ _ _ _ _ _ _ _ _ _ _ _ _ _ _]
      event Timeout {
        n188 = event-data() -> ()  [unwired: 1 in, 1 out]
        n189 = local read "Mode"() -> (w292:T5)
        n190 = case shown="\"Test\"" "Dashboard Tab" {
          tunnel: w295 -> [_ _ w311 _ _]
          tunnel: "TestMode/Automatic/" ("Name Pattern") -> [_ _ w310 _ _]
          tunnel: T21 [{"Operation"=enum."Clear", "Color Box"=14013909}, {"Operation"=enum."Clear", "Color Box"=14013909}, {"Operation"=enum."Clear", "Color Box"=14013909}, {"Operation"=enum."Clear", "Color Box"=14013909}, {"Operation"=enum."Update", "Color Box"=14013909}, {"Operation"=enum."Update", "Color Box"=16777215}, {"Operation"=enum."Clear", "Color Box"=14013909}, {"Operation"=enum."Clear", "Color Box"=14013909}, {"Operation"=enum."Clear", "Color Box"=14013909}] -> [_ _ w303 _ w331]
          tunnel: w292 -> [_ _ w302 _ w330]
          tunnel: u32[] [15790320, 15790320, 15790320, 15790320, 16777215, 16777215, 15790320, 15790320, 15790320] -> [_ _ _ _ w336]
          tunnel: w290 -> [_ _ _ _ w324]
          tunnel: w287 -> [_ w297 _ _ _]
          frame "Custom", Default {
          }
          frame "Basic" {
            n191 = call <vilib>:"WPI_DashboardUpdateNames.vi"("Controls on Tab"=w297) -> ()  [unwired: 11 in]
          }
          frame "Test" {
            w309 = -2 ("Active Item:Row Number")
            n192 = Index Array(array=w303, index=w302) -> (element=w304:T24)
            n193 = Unbundle(w304) -> ("Operation"=w305:enum16{"Update", "Clear"}, "Color Box"=w306:u32)
            n194 = call <vilib>:"NT Read String.vi"("Name"="TestMode/TestName") -> ("String"=w300:string)  [unwired: 9 in, 1 out]
            n195 = call <vilib>:"NT Read and Format Entries as Tree.vi"("Operation"=w305, "Name Pattern"=w310, "Tree Refnum"=w311) -> ()  [unwired: 7 in, 2 out]
            n196 = case shown="\"\"" w300 {
              tunnel: "TestMode/TestProgress" ("Name") -> [w313 _]
              tunnel: "TestMode/TestProgressText" ("Name") -> [w312 _]
              frame Default {
                n197 = call <vilib>:"NT Read Number.vi"("Name"=w313) -> ("Numeric"=w314:dbl)  [unwired: 9 in, 1 out]
                n198 = call <vilib>:"NT Read String.vi"("Name"=w312) -> ("String"=w315:string)  [unwired: 9 in, 1 out]
                n199 = Bundle("Numeric"=w314, "String"=w315) -> (→"Progress":cluster{"Numeric":dbl, "String":string})  [unwired: 1 in]
              }
              frame "" {
                n200 = property on="Progress" class="Clust (strict)"("Visible"=FALSE) -> ()  [unwired: 2 in, 2 out]
                n201 = local write "Test Name"(u16 0) -> ()
              }
            }
            n202 = property on="Test Tree" class="Tree (strict)"("Active Item Row Number"=w309, "ActiveColNum"=w309, "CellBG"=w306, "Active Item Row Number"=-1 ("Active Item:Row Number"), "CellBG"=u32 5789784 ("Color Box")) -> ()  [unwired: 2 in, 2 out]
          }
          frame "Variables" {
            w321 = string[] ["CameraPublisher", "Usage", "DB"]  # Items to initially close
            n203 = First Call?() -> (First Call?: T/F=w322:bool)
            n204 = control-ref of="Tree"() -> (w323:refnum<vi>)
            n205 = Select(t=w321, s=w322, f=string[] []) -> (s? t:f=w319:string[])
            n206 = call <vilib>:"NT Read and Format Entries as Tree.vi"("Tags to  Close"=w319, "Tree Refnum"=w323) -> ()  [unwired: 8 in, 2 out]
          }
          frame "Commands" {
            w332 = u32 5789784 ("Color Box")
            w333 = T25 {"Row"=-1, "Column"=-2} ("Active Cell:Active Cell")
            w335 = T25 {"Row"=-2, "Column"=-2} ("Active Cell:Active Cell")
            n207 = Index Array(array=w336, index=w330) -> (element=w334:u32)
            n208 = Index Array(array=w331, index=w330) -> (element=w329:T24)
            n209 = Unbundle(w329) -> ("Operation"=w328:enum16{"Update", "Clear"})  [unwired: 1 out]
            n210 = local read "Command Selection"() -> (w327:i32)
            n211 = property on="Command Selection" class="MCListbox (strict)"("ActiveCell"=w335, "CellBG"=w334, "ActiveCell"=w333, "CellBG"=w332) -> ()  [unwired: 2 in, 2 out]
            n212 = call <vilib>:"WPI_DashboardUpdate RPC Info.vi"("Operation"=w328) -> ("update"=w326:bool, "commands"=w325:string[][])  [unwired: 9 in]
            n213 = property on="Command Selection" class="MCListbox (strict)"("ItemNames"=w325) -> ()  [unwired: 2 in, 2 out]
            n214 = property on="Command Params" class="Tbl (strict)"("Active Cell"=w335, "Cell BG Color"=w334, "Active Cell"=w333, "Cell BG Color"=w332) -> ()  [unwired: 2 in, 2 out]
            n215 = call <vilib>:"WPI_DashboardUpdate Command Params.vi"("Update"=w326, "NewVal"=w327, "Commands"=w325, "Param Tbl"=w324) -> ()  [unwired: 7 in, 1 out]
          }
        }
        n216 = call <vilib>:"Connextion Info.vi"() -> ("Connected"=→"NT Connection":bool)  [unwired: 10 in, 1 out]
      }
      event "Test Tree": Value Change {
        # "Show appropriate\ncontrols"
        n217 = event-data() -> ("CtlRef"=w341:refnum<vi>, "NewVal"=w339:string)  [unwired: 1 in]
        n218 = call <vilib>:"WPI_UtilitiesGetTreeIOName.vi"("NewVal"=w339, "TreeControl in"=w341) -> ("I/O Name"=w342:string)  [unwired: 9 in]
        n219 = case shown="\"Camera\"" w342 {
          selector: w342 -> [_ w349 _ w371 w380 _]
          tunnel: w339 -> [_ _ w368 w370 _ w387]
          tunnel: cluster{string[]}[] [{["640x480", "320x240", "160x120"]}, {["Auto", "Fixed indoor", "Fixed outdoor 1", "Fixed outdoor 2", "Fixed fluorescent 1", "Fixed fluorescent 2", "Hold current"]}, {["Auto", "Flicker-free 50 Hz", "Flicker-free 60 Hz", "Hold current"]}, {["None", "Prioritize frame rate", "Prioritize image quality"]}, {["Monochrome", "Color"]}] -> [_ _ _ _ _ w386]
          frame Default {
            w344 = FALSE ("Visible")
            w343 = FALSE ("Visible")
            n220 = property on="Motor" class="Clust (strict)"("Visible"=w343) -> ()  [unwired: 2 in, 2 out]
            n221 = property on="Test Ring" class="Ring (strict)"("Visible"=w343) -> ()  [unwired: 2 in, 2 out]
            n222 = property on="Rev/Fwd" class="Clust (strict)"("Visible"=w344) -> ()  [unwired: 2 in, 2 out]
            n223 = property on="On/Off" class="Bool (strict)"("Visible"=w344) -> ()  [unwired: 2 in, 2 out]
            n224 = property on="Test Slider" class="Slide (strict)"("Visible"=w344) -> ()  [unwired: 2 in, 2 out]
          }
          frame "Analog Out", "Motor", "PWM" {
            w350 = FALSE ("Visible")
            n225 = case shown="\"Analog Out\"" w349 {
              tunnel: [1.0 ("Value") -1.0 ("Value") 0.0 ("Value")] -> w348
              tunnel: [255.0 ("Value") 1.0 ("Value") 5.0 ("Value")] -> w347
              tunnel: [128.0 ("Value") 0.0 ("Value") 0.0 ("Value")] -> w346
              tunnel: [64.0 ("Value") 0.5 ("Value") 1.0 ("Value")] -> w345
              frame "PWM" {
              }
              frame "Motor", Default {
              }
              frame "Analog Out" {
              }
            }
            n226 = property on="Motor" class="Clust (strict)"("Visible"=TRUE) -> ()  [unwired: 2 in, 2 out]
            n227 = property on="Value" class="Slide (strict)"("Value"=w346, "Scale.Minimum"=w348, "Scale.Maximum"=w347, "Scale.Increment"=w345) -> ()  [unwired: 2 in, 2 out]
            n228 = property on="On/Off" class="Bool (strict)"("Visible"=w350) -> ()  [unwired: 2 in, 2 out]
            n229 = property on="Test Slider" class="Slide (strict)"("Visible"=w350) -> ()  [unwired: 2 in, 2 out]
            n230 = property on="Test Ring" class="Ring (strict)"("Visible"=w350) -> ()  [unwired: 2 in, 2 out]
            n231 = property on="Rev/Fwd" class="Clust (strict)"("Visible"=w350) -> ()  [unwired: 2 in, 2 out]
          }
          frame "Servo" {
            w366 = FALSE ("Visible")
            n232 = call <vilib>:"NT Read Number.vi"("Name"=w368) -> ("Numeric"=w367:dbl)  [unwired: 9 in, 1 out]
            n233 = property on="Test Slider" class="Slide (strict)"("Visible"=TRUE, "Scale.Maximum"=170.0 ("Scale.Range:Maximum")) -> ()  [unwired: 2 in, 2 out]
            n234 = local write "Test Slider"(w367) -> ()
            n235 = property on="Motor" class="Clust (strict)"("Visible"=w366) -> ()  [unwired: 2 in, 2 out]
            n236 = property on="Rev/Fwd" class="Clust (strict)"("Visible"=w366) -> ()  [unwired: 2 in, 2 out]
            n237 = property on="On/Off" class="Bool (strict)"("Visible"=w366) -> ()  [unwired: 2 in, 2 out]
            n238 = property on="Test Ring" class="Ring (strict)"("Visible"=w366) -> ()  [unwired: 2 in, 2 out]
          }
          frame "Relay", "Solenoid" {
            w369 = FALSE ("Visible")
            n239 = property on="Motor" class="Clust (strict)"("Visible"=w369) -> ()  [unwired: 2 in, 2 out]
            n240 = property on="Test Slider" class="Slide (strict)"("Visible"=w369) -> ()  [unwired: 2 in, 2 out]
            n241 = Search and Replace String(input string=w370, search string="/Value  **", replace string="/Direction") -> (result string=w376:string)  [unwired: 5 in, 3 out]
            n242 = property on="Test Ring" class="Ring (strict)"("Visible"=w369) -> ()  [unwired: 2 in, 2 out]
            n243 = call <vilib>:"NT Read String.vi"("Name"=w376) -> ("String"=w374:string)  [unwired: 9 in, 1 out]
            n244 = Equal?(x="Both directions", y=w374) -> (x = y?=w372:bool)
            n245 = Not(x=w372) -> (.not. x?=w373:bool)
            n246 = property on="Rev/Fwd" class="Clust (strict)"("Visible"=w372) -> ()  [unwired: 2 in, 2 out]
            n247 = property on="On/Off" class="Bool (strict)"("Visible"=w373, "Caption.Text"=w371) -> ()  [unwired: 2 in, 2 out]
          }
          frame "Compressor", "Digital Out" {
            w379 = FALSE ("Visible")
            # "Get direction and finish"
            n248 = property on="Motor" class="Clust (strict)"("Visible"=w379) -> ()  [unwired: 2 in, 2 out]
            n249 = property on="Test Slider" class="Slide (strict)"("Visible"=w379) -> ()  [unwired: 2 in, 2 out]
            n250 = property on="Test Ring" class="Ring (strict)"("Visible"=w379) -> ()  [unwired: 2 in, 2 out]
            n251 = property on="On/Off" class="Bool (strict)"("Visible"=TRUE, "Caption.Text"=w380) -> ()  [unwired: 2 in, 2 out]
            n252 = property on="Rev/Fwd" class="Clust (strict)"("Visible"=FALSE) -> ()  [unwired: 2 in, 2 out]
          }
          frame "Camera" {
            n253 = call <vilib>:"Get Last Path Segment.vi"("String in"=w387) -> ("String out"=w388:string)  [unwired: 10 in]
            n254 = property on="On/Off" class="Bool (strict)"("Visible"=FALSE) -> ()  [unwired: 2 in, 2 out]
            n255 = property on="Motor" class="Clust (strict)"("Visible"=FALSE) -> ()  [unwired: 2 in, 2 out]
            n256 = property on="Rev/Fwd" class="Clust (strict)"("Visible"=FALSE) -> ()  [unwired: 2 in, 2 out]
            n257 = case shown="\"White Balance  **\"" w388 {
              tunnel: w387 -> [w394 w403 w412 w421 w430 _ w436]
              tunnel: w386 -> [w392 w400 w409 w418 w427 _ _]
              frame "Size  **" {
                n258 = Index Array(array=w392) -> (element=w391:cluster{string[]})  [unwired: 1 in]
                n259 = call <vilib>:"NT Read String.vi"("Name"=w394) -> ("String"=w393:string)  [unwired: 9 in, 1 out]
                n260 = Unbundle(w391) -> (w389:string[])
                n261 = Match First String(2:w389, 3:w393) -> (0:w390:i32)  [unwired: 1 out]
                n262 = property on="Test Ring" class="Ring (strict)"("Value"=w390, "Strings []"=w389) -> ()  [unwired: 2 in, 2 out]
                n263 = property on="Test Ring" class="Ring (strict)"("Visible"=TRUE) -> ()  [unwired: 2 in, 2 out]
                n264 = property on="Test Slider" class="Slide (strict)"("Visible"=FALSE) -> ()  [unwired: 2 in, 2 out]
              }
              frame "White Balance  **" {
                n265 = Index Array(array=w400, index=1) -> (element=w401:cluster{string[]})
                n266 = call <vilib>:"NT Read String.vi"("Name"=w403) -> ("String"=w402:string)  [unwired: 9 in, 1 out]
                n267 = Unbundle(w401) -> (w398:string[])
                n268 = Match First String(2:w398, 3:w402) -> (0:w397:i32)  [unwired: 1 out]
                n269 = property on="Test Ring" class="Ring (strict)"("Value"=w397, "Strings []"=w398) -> ()  [unwired: 2 in, 2 out]
                n270 = property on="Test Ring" class="Ring (strict)"("Visible"=TRUE) -> ()  [unwired: 2 in, 2 out]
                n271 = property on="Test Slider" class="Slide (strict)"("Visible"=FALSE) -> ()  [unwired: 2 in, 2 out]
              }
              frame "Exposure  **" {
                n272 = Index Array(array=w409, index=2) -> (element=w410:cluster{string[]})
                n273 = call <vilib>:"NT Read String.vi"("Name"=w412) -> ("String"=w411:string)  [unwired: 9 in, 1 out]
                n274 = Unbundle(w410) -> (w406:string[])
                n275 = Match First String(2:w406, 3:w411) -> (0:w407:i32)  [unwired: 1 out]
                n276 = property on="Test Ring" class="Ring (strict)"("Value"=w407, "Strings []"=w406) -> ()  [unwired: 2 in, 2 out]
                n277 = property on="Test Ring" class="Ring (strict)"("Visible"=TRUE) -> ()  [unwired: 2 in, 2 out]
                n278 = property on="Test Slider" class="Slide (strict)"("Visible"=FALSE) -> ()  [unwired: 2 in, 2 out]
              }
              frame "Exposure Priority  **" {
                n279 = Index Array(array=w418, index=3) -> (element=w419:cluster{string[]})
                n280 = call <vilib>:"NT Read String.vi"("Name"=w421) -> ("String"=w420:string)  [unwired: 9 in, 1 out]
                n281 = Unbundle(w419) -> (w415:string[])
                n282 = Match First String(2:w415, 3:w420) -> (0:w416:i32)  [unwired: 1 out]
                n283 = property on="Test Ring" class="Ring (strict)"("Value"=w416, "Strings []"=w415) -> ()  [unwired: 2 in, 2 out]
                n284 = property on="Test Ring" class="Ring (strict)"("Visible"=TRUE) -> ()  [unwired: 2 in, 2 out]
                n285 = property on="Test Slider" class="Slide (strict)"("Visible"=FALSE) -> ()  [unwired: 2 in, 2 out]
              }
              frame "Color Enable  **" {
                n286 = Index Array(array=w427, index=4) -> (element=w428:cluster{string[]})
                n287 = call <vilib>:"NT Read String.vi"("Name"=w430) -> ("String"=w429:string)  [unwired: 9 in, 1 out]
                n288 = Unbundle(w428) -> (w424:string[])
                n289 = Match First String(2:w424, 3:w429) -> (0:w425:i32)  [unwired: 1 out]
                n290 = property on="Test Ring" class="Ring (strict)"("Value"=w425, "Strings []"=w424) -> ()  [unwired: 2 in, 2 out]
                n291 = property on="Test Ring" class="Ring (strict)"("Visible"=TRUE) -> ()  [unwired: 2 in, 2 out]
                n292 = property on="Test Slider" class="Slide (strict)"("Visible"=FALSE) -> ()  [unwired: 2 in, 2 out]
              }
              frame Default {
                n293 = property on="Test Ring" class="Ring (strict)"("Visible"=FALSE) -> ()  [unwired: 2 in, 2 out]
                n294 = property on="Test Slider" class="Slide (strict)"("Visible"=FALSE) -> ()  [unwired: 2 in, 2 out]
              }
              frame "Brightness  **", "Color Level  **", "Compression  **", "FPS  **", "Sharpness  **" {
                n295 = call <vilib>:"NT Read Number.vi"("Name"=w436) -> ("Numeric"=w435:dbl)  [unwired: 9 in, 1 out]
                n296 = local write "Test Slider"(w435) -> ()
                n297 = property on="Test Slider" class="Slide (strict)"("Visible"=TRUE, "Scale.Maximum"=100.0 ("Scale.Range:Maximum")) -> ()  [unwired: 2 in, 2 out]
                n298 = property on="Test Ring" class="Ring (strict)"("Visible"=FALSE) -> ()  [unwired: 2 in, 2 out]
              }
            }
          }
        }
        n299 = property on="Progress" class="Clust (strict)"("Visible"=FALSE) -> ()  [unwired: 2 in, 2 out]
      }
      event "Test Name": Mouse Enter {
        # "Populate the ring with the list of tests"
        n300 = event-data() -> ()  [unwired: 1 in, 1 out]
        n301 = call <vilib>:"NT Read String Array.vi"("Name"="TestMode/TestList") -> ("String Array"=w444:string[])  [unwired: 9 in, 1 out]
        n302 = Build Array (concatenate)("Select the test to run...", w444) -> (w443:string[])
        n303 = property on="Test Name" class="Ring (strict)"("Strings []"=w443) -> ()  [unwired: 2 in, 2 out]
      }
      event "Test Name": Value Change {
        w446 = FALSE ("Visible")
        # "Tell the robot the test name to run"
        n304 = event-data() -> ("NewVal"=w450:u16)  [unwired: 1 in]
        n305 = property on="Test Name" class="Ring (strict)"() -> ("Strings []"=w451:string[])  [unwired: 2 in, 2 out]
        n306 = local write "Progress"(T6 {"Test Progress"=0, "Test Progress Text"=""} ("Progress")) -> ()
        n307 = Index Array(array=w451, index=w450) -> (element=w449:string)
        n308 = call <vilib>:"NT Write String.vi"("String"=w449, "Name"="TestMode/TestName") -> ()  [unwired: 9 in, 1 out]
        n309 = property on="Progress" class="Clust (strict)"("Visible"=TRUE) -> ()  [unwired: 2 in, 2 out]
        n310 = property on="Motor" class="Clust (strict)"("Visible"=w446) -> ()  [unwired: 2 in, 2 out]
        n311 = property on="Test Slider" class="Slide (strict)"("Visible"=w446) -> ()  [unwired: 2 in, 2 out]
        n312 = property on="On/Off" class="Bool (strict)"("Visible"=w446) -> ()  [unwired: 2 in, 2 out]
        n313 = property on="Rev/Fwd" class="Clust (strict)"("Visible"=w446) -> ()  [unwired: 2 in, 2 out]
        n314 = property on="Test Ring" class="Ring (strict)"("Visible"=w446) -> ()  [unwired: 2 in, 2 out]
      }
      event "Select Auto": Mouse Enter {
        # "Populate the combo box with the list of autonomous options"
        n315 = event-data() -> ()  [unwired: 1 in, 1 out]
        n316 = call <vilib>:"NT Read String Array.vi"("Name"="Auto List") -> ("String Array"=w453:string[])  [unwired: 9 in, 1 out]
        n317 = property on="Select Auto" class="CmbBox"("Strings[]"=w453) -> ()  [unwired: 2 in, 2 out]
      }
      event "Select Auto": Value Change {
        # "User modified the Auto Selection. Write to NT variable so robot knows."
        n318 = event-data() -> ("NewVal"=w456:string)  [unwired: 1 in]
        n319 = call <vilib>:"NT Write String.vi"("String"=w456, "Name"="Auto Selector") -> ()  [unwired: 9 in, 1 out]
      }
      event "Command Selection": Value Change {
        # "Get the params and show in table"
        n320 = event-data() -> ("NewVal"=w462:i32)  [unwired: 1 in]
        n321 = property on="Command Selection" class="MCListbox (strict)"() -> ("ItemNames"=w460:string[][])  [unwired: 2 in, 2 out]
        n322 = call <vilib>:"WPI_DashboardUpdate Command Params.vi"("NewVal"=w462, "Commands"=w460, "Param Tbl"=w461) -> ()  [unwired: 8 in, 1 out]
      }
      event "Execute Command": Value Change {
        # "Started one, Unique ID holds\nresponse"
        n323 = event-data() -> ()  [unwired: 1 in, 1 out]
        n324 = property on="Command Selection" class="MCListbox (strict)"() -> ("ItemNames"=w473:string[][])  [unwired: 2 in, 2 out]
        n325 = Index Array(array=w473, index (row)="Command Selection", index (col)=0) -> (element=w471:string)
        n326 = call <vilib>:"Invoke Commands.vi"("Command Params"="Command Params", "Function Name"=w471) -> ("Params"=w467:u8, "Started"=w466:bool)  [unwired: 7 in, 1 out]
        n327 = Array Subset(array="Command Params", length (row)=w467) -> (w468:string[][])  [unwired: 3 in]
        n328 = Select(t="Executing" ("Cmd Status"), s=w466, f="" ("Cmd Status")) -> (s? t:f=→"Cmd Status":string)
      }
      event "Command Selection": Double Click {
        n329 = event-data() -> ("Row"=w481:i32)  [unwired: 1 in]
        n330 = property on="Command Selection" class="MCListbox (strict)"() -> ("ItemNames"=w484:string[][])  [unwired: 2 in, 2 out]
        n331 = local read "Command Params"() -> (w480:string[][])
        n332 = Index Array(array=w484, index (row)=w481, index (col)=0) -> (element=w482:string)
        n333 = call <vilib>:"Invoke Commands.vi"("Command Params"=w480, "Function Name"=w482) -> ("Params"=w479:u8, "Started"=w474:bool)  [unwired: 7 in, 1 out]
        n334 = Array Subset(array=w480, length (row)=w479) -> (w478:string[][])  [unwired: 3 in]
        n335 = Select(t="Executing" ("Cmd Status"), s=w474, f="" ("Cmd Status")) -> (s? t:f=w475:string)
        n336 = local write "Cmd Status"(w475) -> ()
      }
      event "CheckList": Double Click {
        # "Shift clears all"
        # "Update symbols on the listbox"
        n337 = event-data() -> ("PlatMods.Shift"=w486:bool, "Row"=w488:i32)  [unwired: 1 in]
        n338 = case shown="True" w486 {
          tunnel: w488 -> [w492 _]
          tunnel: 1 -> [w491 _]
          frame False {
            n339 = property on="CheckList" class="LstBox (strict)"() -> ("Item Symbols"=w490:i32[])  [unwired: 2 in, 2 out]
            n340 = Replace Array Subset(array=w490, new element=w491, index=w492) -> (w489:i32[])
            n341 = property on="CheckList" class="LstBox (strict)"("Item Symbols"=w489) -> ()  [unwired: 2 in, 2 out]
          }
          frame True {
            w493 = 0 ("Top Row")
            n342 = property on="CheckList" class="LstBox (strict)"() -> ("Number of Rows"=w495:u32)  [unwired: 2 in, 2 out]
            n343 = Initialize Array(0, w495) -> (w494:i32[])
            n344 = property on="CheckList" class="LstBox (strict)"("Top Row"=w493, "Value"=w493, "Item Symbols"=w494) -> ()  [unwired: 2 in, 2 out]
          }
        }
      }
      event "CheckList": Key Down {
        # "Update symbols on the listbox\nLeft and right keys check and uncheck"
        n345 = event-data() -> ("VKey"=w499:T22)  [unwired: 1 in]
        n346 = case shown="\"Left\", \"Right\"" w499 {
          selector: w499 -> [w504 _]
          tunnel: eventvkey."Left" ("VKey") -> [w502 _]
          frame "Left", "Right" {
            n347 = Equal?(x=w502, y=w504) -> (x = y?=w503:bool)
            n348 = Select(t=0, s=w503, f=1) -> (s? t:f=w505:i32)
            n349 = property on="CheckList" class="LstBox (strict)"() -> ("Item Symbols"=w508:i32[])  [unwired: 2 in, 2 out]
            n350 = Replace Array Subset(array=w508, new element=w505, index="CheckList") -> (w507:i32[])
            n351 = property on="CheckList" class="LstBox (strict)"("Item Symbols"=w507) -> ()  [unwired: 2 in, 2 out]
          }
          frame Default {
          }
        }
      }
      event "Motor.Enable": Value Change {
        # "When the test mode otor enable helper is set, update that\ntree row item's value"
        n352 = event-data() -> ("NewVal"=w514:bool)  [unwired: 1 in]
        n353 = Unbundle("Motor") -> ("Value"=w513:dbl)  [unwired: 1 out]
        n354 = Select(t=w513, s=w514, f=0.0) -> (s? t:f=w511:dbl)
        n355 = call <vilib>:"NT Write Number.vi"("Numeric"=w511, "Name"=w510) -> ()  [unwired: 9 in, 1 out]
      }
      event "Test Slider": Value Change {
        # "When the test mode slider helper is set, update that\ntree row item's value"
        n356 = event-data() -> ("NewVal"=w517:dbl)  [unwired: 1 in]
        n357 = call <vilib>:"NT Write Number.vi"("Numeric"=w517, "Name"=w518) -> ()  [unwired: 9 in, 1 out]
      }
      event "On/Off": Value Change {
        # "When the test mode on/off helper value is set, update that\ntree row item's value"
        n358 = event-data() -> ("NewVal"=w522:bool)  [unwired: 1 in]
        n359 = Boolean To (0,1)(Boolean=w522) -> (0, 1=w521:i16)
        n360 = call <vilib>:"NT Write Number.vi"("Numeric"=w521, "Name"=w520) -> ()  [unwired: 9 in, 1 out]
      }
      event "Rev/Fwd": Value Change {
        # "When the test mode helper value for relays is set, update that\ntree row item's value"
        n361 = event-data() -> ("NewVal.Forward"=w530:bool, "NewVal.Reverse"=w529:bool)  [unwired: 1 in]
        n362 = Boolean To (0,1)(Boolean=w530) -> (0, 1=w526:i16)
        n363 = Boolean To (0,1)(Boolean=w529) -> (0, 1=w528:i16)
        n364 = Negate(x=w528) -> (-x=w527:i16)
        n365 = Add(x=w526, y=w527) -> (x+y=w525:i16)
        n366 = call <vilib>:"NT Write Number.vi"("Numeric"=w525, "Name"=w524) -> ()  [unwired: 9 in, 1 out]
      }
      event "Test Ring": Value Change {
        # "When a test mode helper value is selected from the ring,\nset the tree item's variable to the string value"
        n367 = event-data() -> ("NewVal"=w534:u16)  [unwired: 1 in]
        n368 = property on="Test Ring" class="Ring (strict)"() -> ("Strings []"=w535:string[])  [unwired: 2 in, 2 out]
        n369 = Index Array(array=w535, index=w534) -> (element=w533:string)
        n370 = call <vilib>:"NT Write String.vi"("String"=w533, "Name"=w532) -> ()  [unwired: 9 in, 1 out]
      }
      event "Rec Mode": Value Change {
        # "Update globals for recording mode and path to read log from.\nClear when logging and let NetworkTables set path for vision to\nuse."
        n371 = event-data() -> ("NewVal"=w546:enum32{"Stop", "Record", "Playback"})  [unwired: 1 in]
        n372 = global write "WPI_DashboardLogging Global.vi" "Logging Filename"(path "") -> ()
        n373 = global write "WPI_DashboardLogging Global.vi" "Recording"(w546) -> ()
        n374 = case shown="\"Playback\"" w546 {
          tunnel: w545 -> [_ w548 w557]
          tunnel: [_ _ w556] -> w543
          tunnel: [_ _ w555] -> _
          tunnel: w541 -> [_ _ w553]
          tunnel: cluster{i32, i32} {-250, 170} -> [_ _ w552]
          tunnel: [_ _ T23 {"Image Size"=TRUE, "Image Type"=TRUE, "Pixel Value"=TRUE, "ROI Information"=TRUE, "Zoom Factor"=FALSE} ("Image Information Shown:All Elements")] -> w536
          tunnel: [_ _ TRUE ("Zoom Factor")] -> w537
          tunnel: w539 -> [_ _ w549]
          frame Default {
          }
          frame "Stop", "Record" {
            # "Place Window too"
            n375 = invoke class="VI" method="FP.Close"(reference=w548) -> (reference out=w547:refnum<vi>)  [unwired: 2 in, 2 out]
            n376 = invoke class="VI" method="Abort VI"(reference=w547) -> ()  [unwired: 2 in, 3 out]
          }
          frame "Playback" {
            n377 = call "Open Playback Panel.vi"("Offset"=w552, "DB VI Ref"=w553, "Playback in"=w557) -> ("Playback out"=w554:refnum<vi>)  [unwired: 8 in]
            n378 = register-events(w554, w549) -> (reference out=w556:refnum<event-registration>, error out=w555:errorcluster)  [unwired: 2 in]
          }
        }
        n379 = property on="Camera Image Right" class="ImageControl"("Image Information Shown"=w536, "Image Information Visible"=w537) -> ()  [unwired: 2 in, 2 out]
        n380 = property on="Camera Image" class="ImageControl"("Image Information Shown"=w536, "Image Information Visible"=w537) -> ()  [unwired: 2 in, 2 out]
        n381 = call <vilib>:"WPI_DashboardNT Log FieldName Cache.vi"("Operation"=enum16{"Lookup/Add", "Index", "Clear"}."Clear") -> ()  [unwired: 8 in, 3 out]
      }
      event Panel Close {
        w559 = enum32{"Stop", "Record", "Playback"}."Stop" ("Rec Mode")
        # "Playback window has been closed, abort"
        n382 = event-data() -> ()  [unwired: 1 in, 4 out]
        n383 = local write "Rec Mode"(w559) -> ()
        n384 = global write "WPI_DashboardLogging Global.vi" "Recording"(w559) -> ()
      }
      event Panel Close {
        # "Abort playback window and ourself"
        n385 = event-data() -> ()  [unwired: 1 in, 4 out]
        n386 = invoke class="VI" method="FP.Close"(reference=w563) -> (reference out=w562:refnum<vi>)  [unwired: 2 in, 2 out]
        n387 = invoke class="VI" method="Abort VI"(reference=w562) -> (error out=w561:errorcluster)  [unwired: 2 in, 2 out]
        n388 = invoke class="VI" method="Abort VI"(error in=w561) -> ()  [unwired: 2 in, 3 out]
      }
      event User Event {
        n389 = event-data() -> ("IDs"=w570:cluster{"RPC field ID":u16, "Unique ID":u16}, "String"=w569:string)  [unwired: 1 in]
        n390 = Bundle("IDs"=w570, "String"=w569) -> (w568:T9)  [unwired: 1 in]
        n391 = call <vilib>:"Retrieve RPC Response.vi"("RPC Response"=w568) -> ("Output"=w566:string[][])  [unwired: 10 in]
        n392 = Build Array (concatenate)(w564, w566) -> (w565:string[][])
        n393 = local write "Command Params"(w565) -> ()
        n394 = local write "Cmd Status"("" ("Cmd Status")) -> ()
      }
      event "Tree": Double Click {
        n395 = event-data() -> ("PlatMods"=w576:T26, "Tag"=w573:string)  [unwired: 1 in]
        n396 = Unbundle(w576) -> ("Shift"=w575:bool)  [unwired: 4 out]
        n397 = String Subset(string=w573, length (rest)=1 ("length (rest)")) -> (substring=w572:string)  [unwired: 1 in]
        n398 = Not(x=w575) -> (.not. x?=w574:bool)
        n399 = case shown="\"/\"" w572 {
          tunnel: w573 -> [_ w579]
          tunnel: w574 -> [_ w578]
          frame Default {
          }
          frame "/" {
            n400 = call <vilib>:"NT Update Persistence.vi"("Persistence"=w578, "Name"=w579) -> ()  [unwired: 9 in, 1 out]
          }
        }
      }
    }
  }
  n401 = while {
    tunnel: w67 -> [w581]
    i -> [w584]
    stop <- FALSE stop-if-true
    n402 = Wait (ms)(milliseconds to wait=u32 100) -> ()  [unwired: 1 out]
    n403 = case shown="\"Playback\"" "Rec Mode" {
      tunnel: w584 -> [_ _ w599]
      tunnel: [u32 2829099 ("Base Color") u32 11141120 ("Target Color") w588] -> w580
      frame "Stop", Default {
        # "Reset the color, extra updates don't cost much"
      }
      frame "Record" {
      }
      frame "Playback" {
        # "Playback"
        n404 = Quotient & Remainder(x=w599, y=u32 50 ("milliseconds to wait")) -> (x-y*floor(x/y)=w595:u32)  [unwired: 1 out]
        n405 = Divide(x=w595, y=u32 50 ("milliseconds to wait")) -> (x/y=w592:dbl)
        n406 = Multiply(x=6.283185307179586, y=w592) -> (x*y=w597:dbl)
        n407 = Sine(x=w597) -> (sin(x)=w596:dbl)
        n408 = Absolute Value(x=w596) -> (abs(x)=w589:dbl)
        n409 = call "Interpolate RGB Color.vi"("Proportion"=w589, "Target Color"=u32 30976, "Base Color"=u32 2829099) -> ("Result Color"=w588:u32)  [unwired: 8 in]
      }
    }
    n410 = property class="Pane"(reference=w581, "PaneColor"=w580) -> ()  [unwired: 1 in, 2 out]
  }
  n411 = local write "Dashboard Tab"(T2."Calibration" ("Dashboard Tab")) -> ()
  n412 = property on="On/Off" class="Bool (strict)"("Visible"=w39) -> ()  [unwired: 2 in, 2 out]
  n413 = property on="Motor" class="Clust (strict)"("Visible"=w39) -> ()  [unwired: 2 in, 2 out]
  n414 = property on="Progress" class="Clust (strict)"("Visible"=w39) -> ()  [unwired: 2 in, 2 out]
  n415 = property on="Test Ring" class="Ring (strict)"("Visible"=w39) -> ()  [unwired: 2 in, 2 out]
  n416 = property on="Rev/Fwd" class="Clust (strict)"("Visible"=w39) -> ()  [unwired: 2 in, 2 out]
  n417 = local write "Command Selection"(u16 0 ("milliseconds to wait")) -> ()
  n418 = while {
    tunnel: u16 1741 ("timeout ms (25000)") -> [w601]
    stop <- FALSE stop-if-true
    n419 = TCP Create Listener(10:w601) -> (0:w600:errorcluster, 3:w602:refnum<k5>)  [unwired: 4 in, 1 out]
    n420 = case shown="No Error" w600 {
      selector: w600 -> [w604 _]
      tunnel: w602 -> [w605 _]
      frame No Error {
        n421 = while {
          tunnel: w605 -> [w608]
          tunnel: w604 -> [w607]
          stop <- FALSE stop-if-true
          n422 = TCP Wait On Listener(8:w607, 11:w608) -> (0:w609:errorcluster, 4:w610:refnum<k5>)  [unwired: 2 in, 3 out]
          n423 = local write "TCP"(w610) -> ()
          n424 = case shown="No Error" w609 {
            frame No Error {
            }
            frame Error {
              n425 = Wait (ms)(milliseconds to wait=u32 1000) -> ()  [unwired: 1 out]
            }
          }
        }
      }
      frame Error {
        n426 = Wait (ms)(milliseconds to wait=u32 1000) -> ()  [unwired: 1 out]
      }
    }
  }
  n427 = local write "Command Params"(string[][] [] ("Command Params")) -> ()
  n428 = global write "WPI_DashboardLogging Global.vi" "Recording"(w61) -> ()
  n429 = local write "Rec Mode"(w61) -> ()
  n430 = call <vilib>:"NT Write String.vi"("String"="Select Auto", "Name"="Auto Selector") -> ()  [unwired: 9 in, 1 out]
  n431 = disable-structure shown="Disabled" {
    frame Disabled {
      n432 = feedback #2() -> (w617)  [unwired: 1 in]
      n433 = feedback-in #2() -> (w616)
      n434 = for {
        tunnel: w617 -> [w621]
        tunnel: w616 -> [w622] mode=indexing
        tunnel: [w620] -> w615 mode=indexing
        n435 = Not Equal?(x=w622, y=w621) -> (x != y?=w620:bool)
      }
      n436 = Or Array Elements(Boolean array=w615) -> (logical OR=w614:bool)
      n437 = call "NTSend.vi"() -> ()  [unwired: 12 in]
      n438 = case shown="True" w614 {
        tunnel: w616 -> [_ w619]
        tunnel: "Sent_Data" ("Name") -> [_ w618]
        frame False {
        }
        frame True {
          n439 = call-poly <vilib>:"NT Write Value.vi"("String Array"=w619, "Name"=w618) -> ()  [unwired: 9 in, 1 out]
        }
      }
    }
    frame Enabled {
    }
  }
  n440 = disable-structure shown="Disabled" {
    frame Disabled {
      (unwired) 0
      (unwired) 0
      # "-for good luck"
      n441 = call "IMAQ Create"("Border Size"=0) -> ()  [unwired: 3 in, 3 out]
    }
    frame Enabled {
    }
  }
  n442 = disable-structure shown="Disabled" {
    disable-tunnel: _ -> [w624 _]
    frame Disabled {
      n443 = for {
        tunnel: w624 -> [w628] mode=indexing
        tunnel: [w627] -> _ mode=indexing
        tunnel: [w626] -> _ mode=indexing
        tunnel: [w625] -> _ mode=indexing
        i -> [w639]
        n444 = call <vilib>:"Get Type Information.vi"("variant"=w628) -> ("type"=w641:T27)  [unwired: 6 in, 4 out]
        n445 = call <vilib>:"Get Type Information.vi"("variant"=w628) -> ("type"=w633:T27)  [unwired: 6 in, 4 out]
        n446 = call <vilib>:"Get Type Information.vi"("variant"=w628) -> ("type"=w632:T27)  [unwired: 6 in, 4 out]
        n447 = Equal?(x=w641, y=Data_Type."String") -> (x = y?=w638:bool)
        n448 = Equal?(x=w633, y=Data_Type."Boolean") -> (x = y?=w635:bool)
        n449 = Equal?(x=w632, y=Data_Type."Double Float") -> (x = y?=w630:bool)
        n450 = Select(t=w639, s=w638, f=-1) -> (s? t:f=w627:i32)
        n451 = Select(s=w635, f=-1) -> (s? t:f=w626:i32)  [unwired: 1 in]
        n452 = Select(s=w630, f=-1) -> (s? t:f=w625:i32)  [unwired: 1 in]
      }
    }
    frame Enabled {
    }
  }
